vi "Steuerprogramm-15-07-17.vi"() -> ()   [LabVIEW 2010]
uses:
  Emil/Licor-Steuerung/HAGAR V/Licor-Steuerung/display/GUI_Cluster_sdv.ctl
  Emil/Licor-Steuerung/HAGAR V/Licor-Steuerung/display/GUI_Cluster_Parameter.ctl
  Emil/Licor-Steuerung/HAGAR V/Licor-Steuerung/control/Licor-Commands.ctl
  Emil/Licor-Steuerung/HAGAR V/Licor-Steuerung/control/Licor-Parameter.ctl
  Emil/Licor-Steuerung/LicorLI7000/conventions/Licor-Source.ctl
  Emil/Licor-Steuerung/HAGAR V/Licor-Steuerung/control/Licor-Pump.ctl
  Emil/Licor-Steuerung/HAGAR V/Licor-Steuerung/display/GUI_Cluster_Graph.ctl
  Emil/Licor-Steuerung/HAGAR V/Licor-Steuerung/control/Licor-Sequences.ctl
  <vilib>/rvi/interface/nirviMethod/nirviMethod.xnode
  C:/Users/HAGAR-IV/Desktop/Zeugs/markus/version feb 2012/FPGA Bitfiles/pertrasgcfpga2_FPGATarget_FPGA-Programm-05_A75D3647.lvbitx
  C:/Users/HAGAR-IV/Desktop/Zeugs/Johnny/pertrasgc fpga/FPGA-Programm-05-17.vi
  <vilib>/rvi/interface/common/niFpgaNodeNameForErrorReporting.ctl
  <vilib>/rvi/errors/niLvFpgaWhatHappensToTopLevelVI.ctl
  <vilib>/rvi/interface/nirviReadWriteControl/nirviReadWriteControl.xnode
  <vilib>/rvi/interface/nirviCloseFPGA/nirviCloseFPGA.xnode
  GVProbenvol.vi
  GVZeitenZyklen.vi
  GVECDs.vi
  GVZwangs.vi
  GVMethodenwechsel.vi
  GVTrapsMachs.vi
  GVHK1Hz.vi
  GVAIs.vi
  gvbooleschRT.vi
  GVMetavariablen.vi
  GVVentilposition.vi
  GVHorstSP.vi
  GVMWHorst.vi
  GVHeizenLH.vi
  <vilib>/Utility/error.llb/Error Cluster From Error Code.vi
  <vilib>/rvi/errors/niLvFpgaAdjustHostInterfaceError.vi
  GVaktuelleTDMS.vi
  Emil/Licor-Steuerung/HAGAR V/Licor-Steuerung/control/Emulate Licor output GV.vi
  GVChroms.vi
  GVZwangsMPV.vi
  <vilib>/FPGAPlugInAG/cRIO-9114/niLvFpga_Close_cRIO-9114.vi
  NiFpgaLv.dll
  Emil/Licor-Steuerung/HAGAR V/Licor-Steuerung/Licor-Steuerung.lvlib
  <vilib>/NI_Real-Time Target Support.lvlib
  Emil/Licor-Steuerung/LicorLI7000/LicorLI7000.lvlib
panel:
  in  "Zyklus":enum16{"Mod0", "Mod1", "Mod2A", "Mod2B"}(ring)=enum."Mod1"
  in  "am Ende benutzen":bool
  in  "Methode speichern":bool
  out "ZyklusNummernGesamt":i32[](array[numeric])
  in  "veränderte Methode benutzen":bool
  in  "Methode verändern":bool
  out "ZyklusNummern":i32[](array[numeric])
  out "Big Ben, Methodenzeit, Zykluszeit0, Zykluszeit1, Zykluszeit2A, Zykluszeit2B":i32[](array[numeric])
  in  "global stop RT":bool
  in  "Methode":i32(ring) items=["Bedingsmethode", "Startmethode", "Meßmodus", "Shut-up-Methode", "Test", "HAG2 1/2", "Startmethode", "HAG2 1/2 Aufwärmen", "LicorDruckProfil1", "LicorDruckProfil2", "LicorDruckProfil0", "LicorDruckProfil3", "Kalibration-Meßmodus", "Kalibration-Meßmodus-II", "Kalibration-MesmodusIII", "Kalibration-Messmodus-IV", "Kalibration-ECD", "", "Kalibration-ECD-Blank", "Linearitätstest MS"]
  in  "Registerkarte":T1(tab)
  out "SHOK?":bool[](array[boolean])
  out "schnelle Heizungen":string[](array[string])
  out "schnelle Heizungen":dbl[](array[numeric])
  out "HorstOK?":bool[](array[boolean])
  out "AIs3OK?":bool[](array[boolean])
  out "AIs1OK?":bool[](array[boolean])
  out "AIs1":dbl[](array[numeric])
  out "AIs1":string[](array[string])
  out "AIs2":string[](array[string])
  out "AIs3":string[](array[string])
  out "AIs2":dbl[](array[numeric])
  out "AIs3":dbl[](array[numeric])
  out "Metavariablen":string[](array[string])
  out "MVWerte":dbl[](array[numeric])
  out "MWHorst":dbl[](array[numeric])
  out "HorstRegler":string[](array[string])
  out "AIs2OK?":bool[](array[boolean])
  out "Ventilposition":i32=1 min=1 max=6 step=1
  out "MVOK?":bool[](array[boolean])
  out "CPU Total (%)":dbl
  in  "MVFixwert":dbl[](array[numeric])
  in  "MVFix?":bool[](array[boolean])
  in  "LH-Gruppe":bool[](array[boolean])=[FALSE, FALSE, FALSE, FALSE, FALSE, FALSE, FALSE, FALSE, FALSE, FALSE, FALSE, FALSE]
  out "LangsameHeizungen":string[](array[string])
  out "Housekeeping1":cluster{dbl[], dbl[]}(graph)
  in  "Zeitachse1":i32(ring)=1 items=["Zykluszeit [s] Mod0", "Zykluszeit [s] Mod1", "Zykluszeit [s] Mod2A", "Zykluszeit [s] Mod2B"]
  in  "dargestellte Größe 1":i32(ring)=1 items=["T1-Spare1", "T1-Spare2", "T1-StirlingKühlkopf [°C]", "T1-PreCol1 [°C]", "T1-PreCol2 [°C]", "T1-MainCol1a [°C]", "T1-MainCol1b [°C]", "T1-MainCol2a [°C]", "T1-MainCol2b [°C]", "T1-BronkhorstUntena [°C]", "T1-BronkhorstUntenb [°C]", "T1-BronkhorstObena [°C]", "T1-BronkhorstObenb [°C]", "T1-2Pos1B [°C]", "T1-Spare9", "T1-2Pos1A [°C]", "T1-Spare10", "T1-TurboPump [°C]", "T1-StirlingPlatine [°C]", "T1-Spare5", "T1-Spare6", "T1-Spare7", "T1-Inlet [°C]", "F1-MFM-Spare", "F1-MFM0D [mL]", "P1-HeliumHP [bara]", "P1-HeliumLP [bara]", "P1-PumpVordruck [mbara]", "TurboSpeed", "I1-MS-AC [A]", "I1-Trap1 [A]", "I1-Trap2 [A]", "T2-ECD1a", "T2-ECD1b", "T2-ECD2a", "T2-ECD2b", "T2-Col1a", "T2-Col1b", "T2-Col2a", "T2-Col2b", "T2-Spare1", "T2-Spare2", "T2-Spare3", "T2-Spare4", "T2-Spare5", "T2-Spare6", "T2-Spare7", "F2-MFM2A", "F2-MFM2B", "F2-MFM2C", "P2-N2O_HP", "P2-N2O_LP", "P2-CO2_HP", "P2-CO2_LP", "AI-Spare1", "FL-MFM1000mL", "AI-Spare3", "AI-Spare4", "StirlingAlarm", "StirlingEmerg.", "AI-Spare7", "AI-Spare8", "AI-Spare9", "FL-MFM30mL", "T0-DC/DC5", "I0-24V_M0", "I0-48V_M1", "I0-24V_M1", "I0-28V_M2", "T0-Spare3", "T0-Spare2", "T0-Spare4", "T0-DC/DC7", "I0-20V_Laptop", "I0-28V_M1", "I0-24V_M2", "I0-12V_Licor", "T0-Spare1", "T0-Drier", "T0-Spare5", "F0-MFM0A [L]", "TL-Licor_a", "P0-Span-HP", "P0-spare1", "P0-Stickstoff-LP", "P0-Helium-LP", "P0-Cal-HP", "P0-P9Tavco[bar]", "F0-MFM0B [L]", "TL-Licor_b", "P0-Span-LP", "P0-spare2", "P0-Stickstoff-HP", "P0-Helium-HP", "P0-Cal-LP", "F0-MFM3", "Trap1 [°C]", "Trap2 [°C]", "PreCol1 [°C]", "PreCol2 [°C]", "MainCol1 [°C]", "MainCol2 [°C]", "PrC0 [bara]", "PrC0-Licor [bara]", "PrC1-Säule1 [bara]", "PrC1-Säule2 [bara]", "MFC1-Sample [ml/min]", "PrC1-BackFlush1 [bara]", "PrC1-BackFlush2 [bara]", "MFC1-Reaktant [l/min]", "MFC2A[ml/min]", "MFC2B[ml/min]", "MFC2C[ul/min]", "PrC2A[bara]", "MFC2D[ml/min]", "MFC2E[ml/min]", "PrC2B[bara]"]
  out "Housekeeping2":cluster{dbl[], dbl[]}(graph)
  in  "Zeitachse2":i32(ring)=1 items=["Zykluszeit [s] Mod0", "Zykluszeit [s] Mod1", "Zykluszeit [s] Mod2A", "Zykluszeit [s] Mod2B"]
  in  "dargestellte Größe 2":i32(ring)=1 items=["T1-Spare1", "T1-Spare2", "T1-StirlingKühlkopf [°C]", "T1-PreCol1 [°C]", "T1-PreCol2 [°C]", "T1-MainCol1a [°C]", "T1-MainCol1b [°C]", "T1-MainCol2a [°C]", "T1-MainCol2b [°C]", "T1-BronkhorstUntena [°C]", "T1-BronkhorstUntenb [°C]", "T1-BronkhorstObena [°C]", "T1-BronkhorstObenb [°C]", "T1-2Pos1B [°C]", "T1-Spare9", "T1-2Pos1A [°C]", "T1-Spare10", "T1-TurboPump [°C]", "T1-StirlingPlatine [°C]", "T1-Spare5", "T1-Spare6", "T1-Spare7", "T1-Inlet [°C]", "F1-MFM-Spare", "F1-MFM0D [mL]", "P1-HeliumHP [bara]", "P1-HeliumLP [bara]", "P1-PumpVordruck [mbara]", "TurboSpeed", "I1-MS-AC [A]", "I1-Trap1 [A]", "I1-Trap2 [A]", "T2-ECD1a", "T2-ECD1b", "T2-ECD2a", "T2-ECD2b", "T2-Col1a", "T2-Col1b", "T2-Col2a", "T2-Col2b", "T2-Spare1", "T2-Spare2", "T2-Spare3", "T2-Spare4", "T2-Spare5", "T2-Spare6", "T2-Spare7", "F2-MFM2A", "F2-MFM2B", "F2-MFM2C", "P2-N2O_HP", "P2-N2O_LP", "P2-CO2_HP", "P2-CO2_LP", "AI-Spare1", "FL-MFM1000mL", "AI-Spare3", "AI-Spare4", "StirlingAlarm", "StirlingEmerg.", "AI-Spare7", "AI-Spare8", "AI-Spare9", "FL-MFM30mL", "T0-DC/DC5", "I0-24V_M0", "I0-48V_M1", "I0-24V_M1", "I0-28V_M2", "T0-Spare3", "T0-Spare2", "T0-Spare4", "T0-DC/DC7", "I0-20V_Laptop", "I0-28V_M1", "I0-24V_M2", "I0-12V_Licor", "T0-Spare1", "T0-Drier", "T0-Spare5", "F0-MFM0A [L]", "TL-Licor_a", "P0-Span-HP", "P0-spare1", "P0-Stickstoff-LP", "P0-Helium-LP", "P0-Cal-HP", "P0-P9Tavco[bar]", "F0-MFM0B [L]", "TL-Licor_b", "P0-Span-LP", "P0-spare2", "P0-Stickstoff-HP", "P0-Helium-HP", "P0-Cal-LP", "F0-MFM3", "Trap1 [°C]", "Trap2 [°C]", "PreCol1 [°C]", "PreCol2 [°C]", "MainCol1 [°C]", "MainCol2 [°C]", "PrC0 [bara]", "PrC0-Licor [bara]", "PrC1-Säule1 [bara]", "PrC1-Säule2 [bara]", "MFC1-Sample [ml/min]", "PrC1-BackFlush1 [bara]", "PrC1-BackFlush2 [bara]", "MFC1-Reaktant [l/min]", "MFC2A[ml/min]", "MFC2B[ml/min]", "MFC2C[ul/min]", "PrC2A[bara]", "MFC2D[ml/min]", "MFC2E[ml/min]", "PrC2B[bara]"]
  out "Detektor 2":cluster{dbl[], dbl[]}[](graph)
  in  "Detektor":i32(ring) items=["ECD1", "ECD2"]
  in  "HK1YMin":dbl
  in  "HK1YMax":dbl=100.0
  in  "HK2YMin":dbl
  in  "HK2YMax":dbl=100.0
  in  "DetYMin":dbl
  in  "DetYMax":dbl=100.0
  in  "NeuerRefstrom":bool
  in  "RefStromECD1":i16=800 min=0 max=2500 step=1
  in  "RefStromECD2":i16=2100 min=0 max=2500 step=1
  out "schnelleAnzeige":cluster{dbl[], dbl[]}(graph)
  in  "TafelWischen!":bool
  in  "dargestellte Größe 3":i32(ring)=1 items=["Trap1 [°C]", "Trap2 [°C]", "PreCol1 [°C]", "PreCol2 [°C]", "MainCol1 [°C]", "MainCol2 [°C]", "PrC0 [bara]", "PrC0-Licor [bara]", "PrC1-Säule1 [bara]", "PrC1-Säule2 [bara]", "MFC1-Sample [ml/min]", "PrC1-BackFlush1 [bara]", "PrC1-BackFlush2 [bara]", "MFC1-Reaktant [l/min]", "MFC2A[ml/min]", "MFC2B[ml/min]", "MFC2C[ul/min]", "PrC2A[bara]", "MFC2D[ml/min]", "MFC2E[ml/min]", "PrC2B[bara]"]
  in  "An/Aus":bool
  in  "Registerkarte 2":T2(tab)
  in  "GUI_Cluster_Graph":T3={"time (global)"=0.0, "command queue"=[], "Rohdaten"=[], "Graph"={"X"=[], "Y"=[]}, "Manuelle Steuerung"={"Sequenz"=enum."test", "Manuelle Steuerung An/Aus"=FALSE}, "Sequenz out"={"sequence"=enum."WAIT", "Zeitpunkt next"=0.0, "delta t"=0.0}} caption="Cluster" {"Sequenz out"."Zeitpunkt next" format="%<%H:%M:%S%3u>T"; "time (global)" format="%<%H:%M:%S%3u\n%m/%d/%y>T"}
  in  "GUI_Cluster_Parameter":T5={"warmup (sequence)"=[{"time"=60, "Enum"=enum."wait"}], "calibrate S (sequence)"=[{"time"=60, "Enum"=enum."wait"}, {"time"=2, "Enum"=enum."getCalibrationParameter"}, {"time"=8, "Enum"=enum."calibration-S-CO2"}, {"time"=2, "Enum"=enum."getCalibrationParameter"}], "calibrate Z (sequence)"=[{"time"=60, "Enum"=enum."wait"}, {"time"=2, "Enum"=enum."getCalibrationParameter"}, {"time"=8, "Enum"=enum."calibration-Z-H2O"}, {"time"=2, "Enum"=enum."getCalibrationParameter"}, {"time"=8, "Enum"=enum."calibration-Z-CO2"}, {"time"=2, "Enum"=enum."getCalibrationParameter"}], "initialize (sequence)"=[{"time"=30, "Enum"=enum."wait"}, {"time"=2, "Enum"=enum."setPumpSlow"}, {"time"=2, "Enum"=enum."setPumpMedium"}, {"time"=2, "Enum"=enum."setPumpFast"}, {"time"=10, "Enum"=enum."initialize"}, {"time"=4, "Enum"=enum."getCalibrationParameter"}, {"time"=2, "Enum"=enum."resetH2O"}, {"time"=4, "Enum"=enum."resetCO2"}, {"time"=4, "Enum"=enum."getCalibrationParameter"}, {"time"=2, "Enum"=enum."setZeroParameter"}, {"time"=4, "Enum"=enum."getCalibrationParameter"}, {"time"=2, "Enum"=enum."setReference"}, {"time"=4, "Enum"=enum."getLicorTime"}, {"time"=5, "Enum"=enum."getInfo"}], "Licor-parameter"={"CO2 ref"=378.15, "CO2 span"=401.67, "H2O ref"=0.0, "H2O span"=0.0, "Zi"=1.2, "Zt"=6.494e-05, "Zm"=0.0, "S"=1.34, "Temp [C]"=45.0, "Pressure [hPa]"=1050.0, "Licor-Sources"=["CO2A W", "CO2B W", "H2OA W", "H2OB W", "T C", "T V", "P kPa", "P V", "RH %"], "Licor-Pump"="Off", "Zeitstempel"=timestamp(0 s since 1904-01-01)}} {"Licor-parameter"."Pressure [hPa]" format="%_5g"; "Licor-parameter"."Temp [C]" format="%.2f"; "Licor-parameter"."CO2 ref" format="%.2f"; "Licor-parameter"."CO2 span" format="%.2g"; "Licor-parameter"."H2O ref" format="%.2g"; "Licor-parameter"."H2O span" format="%.2g"; "Licor-parameter"."Zt" format="%#_4g"}
  in  "GUI_Cluster_sdv":T10={"Graph_sdv"={"X"=[], "Y"=[]}, "Breite"=20, "Berechnen"=FALSE, "residue"=0.0} {"residue" format="%_6g"}
  in  "VISA resource name":refnum<visa-resource-name>="ASRL1::INSTR" caption="VISA-Ressourcenname"
  out "TDMSwriteECD":errorcluster
  out "AIsFIFOread":errorcluster
  out "MWTrapsMachs":errorcluster
  out "TDMSwriteHK":errorcluster
  out "TDMScloseHK":errorcluster
  out "TDMSopenHK":errorcluster
  out "TDMScloseECD2":errorcluster
  out "TDMSopenECD2":errorcluster
  out "TDMScloseECD1":errorcluster
  out "TDMSopenECD1":errorcluster
  out "FIFOwriteRS485":errorcluster
  out "SerielleKomm.":errorcluster
  out "LH":errorcluster
  out "Zyklus":errorcluster
  out "ECD1dataBackup":errorcluster
  out "ECD2dataBackup":errorcluster
  # "Zyklen:   ===>>"
  # "MS"
  # "ECD1"
  # "ECD2"
  # "Zykluszeiten:   ===>>"
  # "MS"
  # "ECD1"
  # "ECD2"
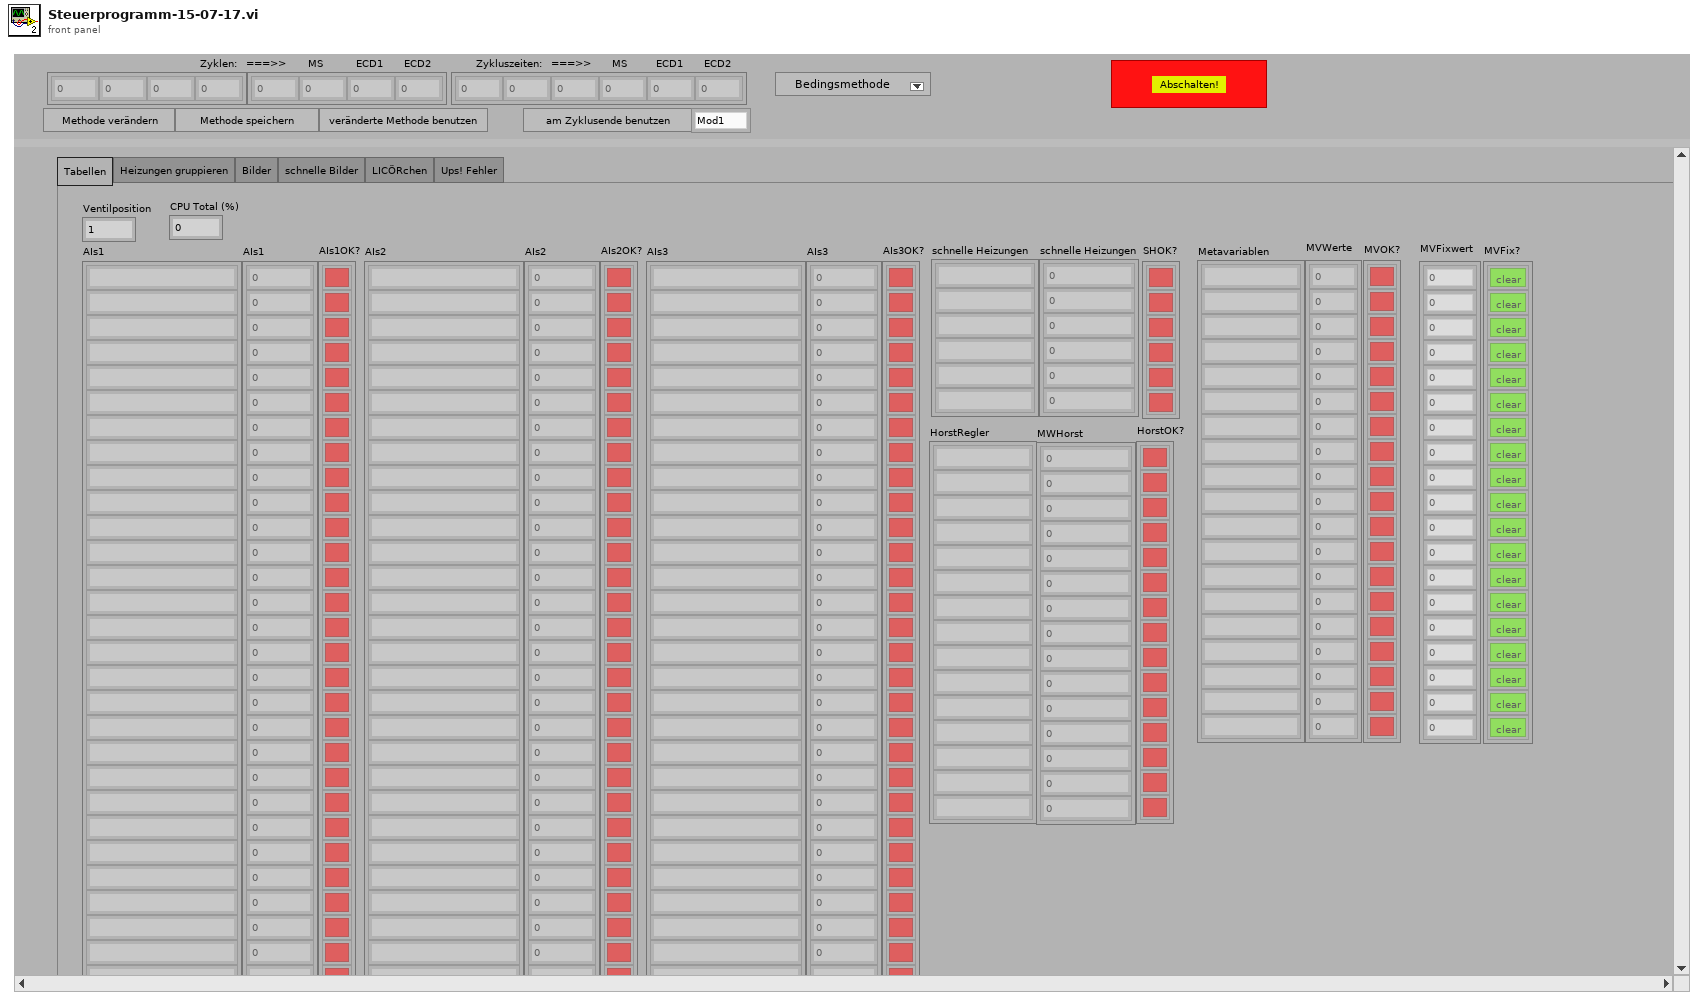
[diagram p1: front panel]
types:
  T1 = enum32{"Tabellen", "Heizungen gruppieren", "Bilder", "schnelle Bilder", "LICÖRchen", "Ups! Fehler"}
  T2 = enum32{"Graph", "Parameter / Sequenzen", "sdv", "debug"}
  T3 = typedef "Licor-Steuerung.lvlib/GUI_Cluster_Graph.ctl" = cluster{"time (global)":dbl, "command queue":cluster{"Zeit [s]":i32, "Befehl":string}[], "Rohdaten":string[], "Graph":cluster{"X":dbl[], "Y":dbl[]}, "Manuelle Steuerung":cluster{"Sequenz":T4, "Manuelle Steuerung An/Aus":bool}, "Sequenz out":cluster{"sequence":T4, "Zeitpunkt next":dbl, "delta t":dbl}}
  T4 = typedef "Licor-Steuerung.lvlib/Licor-Sequences.ctl" = enum16{"test", "WAIT", "warmup", "initialize", "calibrate Z", "calibrate S"}
  T5 = typedef "Licor-Steuerung.lvlib/GUI_Cluster_Parameter.ctl" = cluster{"warmup (sequence)":cluster{"time":i32, "Enum":T6}[], "calibrate S (sequence)":cluster{"time":i32, "Enum":T6}[], "calibrate Z (sequence)":cluster{"time":i32, "Enum":T6}[], "initialize (sequence)":cluster{"time":i32, "Enum":T6}[], "Licor-parameter":T7}
  T6 = typedef "Licor-Steuerung.lvlib/Licor-Commands.ctl" = enum16{"wait", "initialize", "resetCO2", "resetH2O", "getReference", "setReference", "calibration-Z-CO2", "calibration-Z-H2O", "calibration-S-CO2", "calibration-S-H2O", "getCalibrationParameter", "setZeroParameter", "setLicorTime", "getLicorTime", "setPumpFlowrate", "setPumpSlow", "setPumpMedium", "setPumpFast", "getInfo"}
  T7 = typedef "Licor-Steuerung.lvlib/Licor-Parameter.ctl" = cluster{"CO2 ref":dbl, "CO2 span":dbl, "H2O ref":dbl, "H2O span":dbl, "Zi":dbl, "Zt":dbl, "Zm":dbl, "S":dbl, "Temp [C]":dbl, "Pressure [hPa]":dbl, "Licor-Sources":T8[], "Licor-Pump":T9, "Zeitstempel":timestamp}
  T8 = typedef "LicorLI7000.lvlib/Licor-Source.ctl" = string
  T9 = typedef "Licor-Steuerung.lvlib/Licor-Pump.ctl" = string
  T10 = typedef "Licor-Steuerung.lvlib/GUI_Cluster_sdv.ctl" = cluster{"Graph_sdv":cluster{"X":dbl[], "Y":dbl[]}, "Breite":i32, "Berechnen":bool, "residue":dbl}
  T11 = cluster{"Zykluslängen [s]":dbl[], "ZeitpktDIOsMod0":dbl[], "ZeitpktDIOsMod1":dbl[], "ZeitpktDIOsMod2A":dbl[], "ZeitpktDIOsMod2B":dbl[], "DIOsSPMod0":bool[][], "DIOsSPMod1":bool[][], "DIOsSPMod2A":bool[][], "DIOsSPMod2B":bool[][], "Mod0HorstZeitpkt":dbl[], "Mod1HorstZeitpkt":dbl[], "Mod2AHorstZeitpkt":dbl[], "Mod2BHorstZeitpkt":dbl[], "HorstSPMod0":dbl[][], "HorstSPMod1":dbl[][], "HorstSPMod2A":dbl[][], "HorstSPMod2B":dbl[][], "LHSetpoints":dbl[], "LHHeizen?":bool[], "ZPktFPGABoolesch":dbl[], "FPGABoolesch":bool[][], "ZeitpktFPGAPID":dbl[], "FPGAPID":cluster{"d0":fxp<+/-,18,18>, "d1":fxp<+/-,21,21>}[][], "ZeitpktFPGAFixp":dbl[], dbl[][], "t_PreMach1":dbl[], "T_PreMach1":dbl[], "t_PreMach2":dbl[], "T_PreMach2":dbl[], "PIDs für \"träge\" Heizungen":cluster{"proportional gain (Kc)":dbl, "integral time (Ti, min)":dbl, "derivative time (Td, min)":dbl}[], "Zwangsbedingungen":dbl[][], "Dateien fürs MS schicken?":bool, "ZeitpunkteMPV":dbl[], "SPMPV":i32[], "ZeitpktMS-1":dbl, "ZeitpktMS-2":dbl, "Int.Start1":dbl, "Int.Stop1":dbl, "Int.Start2":dbl, "Int.Stop2":dbl, "Methodenname":string, "t_MainMach1":dbl[], "T_MainMach1":dbl[], "t_MainMach2":dbl[], "T_MainMach2":dbl[]}[]
  T12 = cluster{"DIOsMod0Nr":i32[], "DIOsMod1Nr":i32[], "DIOsMod2ANr":i32[], "DIOsMod2BNr":i32[], "AIsLH":i32[], "AnzahlRegler/Modul":i32[], "Regler für den Probenfluß":i32, "SPvorgebenMod0":string[], "SPvorgebenMod1":string[], "SPvorgebenMod2A":string[], "SPvorgebenMod2B":string[], "MWAntwortMod0":string[], "MWAntwortMod1":string[], "MWAntwortMod2A":string[], "MWAntwortMod2B":string[], "FaktorMod0":dbl[], "FaktorMod1":dbl[], "FaktorMod2A":dbl[], "FaktorMod2B":dbl[], "MWabfragenMod0":string[], "MWabfragenMod1":string[], "MWabfragenMod2A":string[], "MWabfragenMod2B":string[], "Modul1/AI koeff":dbl[][], "Modul2/AI koeff":dbl[][], "Modul3/AI koeff":dbl[][], "Traps/MachsKoeff T(R)":dbl[][], "Modul1/AIsNamen":string[], "Modul2/AIsNamen":string[], "Modul3/AIsNamen":string[], "DIOsMod0Name":string[], "DIOsMod1Name":string[], "DIOsMod2AName":string[], "DIOsMod2BName":string[], "ReglerNameMod0":string[], "ReglerNameMod1":string[], "ReglerNameMod2A":string[], "ReglerNameMod2B":string[], "Startmethode":i32, "Dateiordner Housekeeping":path, "Dateiname Housekeeping":string, "DateiordnerECD1":path, "DateinameECD1":string, "DateiordnerECD2":path, "DateinameECD2":string, "LangsameHeizungen":string[], "ModuleLH":i32[], "Metavariablen":string[], "Modul1/AI sicherer Bereich":dbl[][], "Modul2/AI sicherer Bereich":dbl[][], "Modul3/AI sicherer Bereich":dbl[][], "Traps/Machs sicherer Bereich":dbl[][], "ReglerMod0 sicherer Bereich":dbl[][], "ReglerMod1 sicherer Bereich":dbl[][], "ReglerMod2A sicherer Bereich":dbl[][], "ReglerMod2B sicherer Bereich":dbl[][], "Metavariablen grüner Bereich":dbl[][], "Traps/MachsKoeff R(U)":dbl[][], "LHGruppe":bool[]}
  T13 = enum16{"open", "replace", "create", "open or create", "replace or create", "replace or create with confirmation"}
  T14 = typedef "niFpgaNodeNameForErrorReporting.ctl" = enum16{"Open FPGA VI Reference", "Read/Write Control", "Invoke Method: Abort", "Invoke Method: Acknowledge IRQ", "Invoke Method: Download", "Invoke Method: FIFO.Configure", "Invoke Method: FIFO.Read", "Invoke Method: FIFO.Start", "Invoke Method: FIFO.Stop", "Invoke Method: FIFO.Write", "Invoke Method: Reset", "Invoke Method: Run", "Invoke Method: Wait on IRQ", "Close FPGA VI Reference"}
  T15 = typedef "niLvFpgaWhatHappensToTopLevelVI.ctl" = enum16{"top level VI scripted behind XNode", "top level VI inlined behind XNode"}
  T16 = cluster{"Zyklus1":i32, "Zeitachse1":i32, "dargestellte Größe 1":i32, "Zyklus2":i32, "Zeitachse2":i32, "dargestellte Größe 2":i32}
  T17 = cluster{"DIOsMod0Name":string[], "DIOsMod1Name":string[], "DIOsMod2AName":string[], "DIOsMod2BName":string[], "ReglerNameMod0":string[], "ReglerNameMod1":string[], "ReglerNameMod2A":string[], "ReglerNameMod2B":string[], "LangsameHeizungen":string[]}
  T18 = cluster{"Zykluslängen [s]":dbl[], "ZeitpktDIOsMod0":dbl[], "ZeitpktDIOsMod1":dbl[], "ZeitpktDIOsMod2A":dbl[], "ZeitpktDIOsMod2B":dbl[], "DIOsSPMod0":bool[][], "DIOsSPMod1":bool[][], "DIOsSPMod2A":bool[][], "DIOsSPMod2B":bool[][], "Mod0HorstZeitpkt":dbl[], "Mod1HorstZeitpkt":dbl[], "Mod2AHorstZeitpkt":dbl[], "Mod2BHorstZeitpkt":dbl[], "HorstSPMod0":dbl[][], "HorstSPMod1":dbl[][], "HorstSPMod2A":dbl[][], "HorstSPMod2B":dbl[][], "LHSetpoints":dbl[], "LHHeizen?":bool[], "ZPktFPGABoolesch":dbl[], "FPGABoolesch":bool[][], "ZeitpktFPGAPID":dbl[], "FPGAPID":cluster{"d0":fxp<+/-,18,18>, "d1":fxp<+/-,21,21>}[][], "ZeitpktFPGAFixp":dbl[], dbl[][], "t_PreMach1":dbl[], "T_PreMach1":dbl[], "t_PreMach2":dbl[], "T_PreMach2":dbl[], "PIDs für \"träge\" Heizungen":cluster{"proportional gain (Kc)":dbl, "integral time (Ti, min)":dbl, "derivative time (Td, min)":dbl}[], "Zwangsbedingungen":dbl[][], "Dateien fürs MS schicken?":bool, "ZeitpunkteMPV":dbl[], "SPMPV":i32[], "ZeitpktMS-1":dbl, "ZeitpktMS-2":dbl, "Int.Start1":dbl, "Int.Stop1":dbl, "Int.Start2":dbl, "Int.Stop2":dbl, "Methodenname":string, "t_MainMach1":dbl[], "T_MainMach1":dbl[], "t_MainMach2":dbl[], "T_MainMach2":dbl[]}
  T19 = cluster{"Modul1/AI sicherer Bereich":dbl[][], "Modul2/AI sicherer Bereich":dbl[][], "Modul3/AI sicherer Bereich":dbl[][], "Traps/Machs sicherer Bereich":dbl[][], dbl[][], "Metavariablen grüner Bereich":dbl[][]}
  T20 = cluster{"created path":path, "created path":path}
  T21 = cluster{"created path":path, "created path":path, "created path":path, "Dateiname Housekeeping":string, "DateinameECD1":string, "DateinameECD2":string, "tdms0":refnum<k34>, "tdms1":refnum<k34>, "tdms0":refnum<k34>, "tdms1":refnum<k34>, "tdms0":refnum<k34>, "tdms1":refnum<k34>}
  T22 = cluster{"d0":fxp<+/-,18,18>, "d1":fxp<+/-,21,21>}[][]
  T23 = cluster{"proportional gain (Kc)":dbl, "integral time (Ti, min)":dbl, "derivative time (Td, min)":dbl}[]
  T24 = cluster{cluster{"ZeitpktDIOsMod2B":dbl[]}[], cluster{"DIOsSPMod2B":bool[][]}[], cluster{"Mod2BHorstZeitpkt":dbl[]}[], cluster{"HorstSPMod2B":dbl[][]}[], "LHHeizen?":bool[], "ZPktFPGABoolesch":dbl[], "FPGABoolesch":bool[][], "ZeitpktFPGAPID":dbl[], "FPGAPID":cluster{"d0":fxp<+/-,18,18>, "d1":fxp<+/-,21,21>}[][], "ZeitpktFPGAFixp":dbl[], dbl[][], "t_PreMach1":dbl[], "T_PreMach1":dbl[], "t_PreMach2":dbl[], "T_PreMach2":dbl[], "ZeitpunkteMPV":dbl[], "SPMPV":i32[], "t_MainMach1":dbl[], "T_MainMach1":dbl[], "t_MainMach2":dbl[], "T_MainMach2":dbl[]}
  T25 = cluster{"Zykluslängen [s]":dbl[], "ZeitpktDIOsMod0":dbl[], "ZeitpktDIOsMod1":dbl[], "ZeitpktDIOsMod2A":dbl[], "ZeitpktDIOsMod2B":dbl[], "DIOsSPMod0":bool[][], "DIOsSPMod1":bool[][], "DIOsSPMod2A":bool[][], "DIOsSPMod2B":bool[][], "Mod0HorstZeitpkt":dbl[], "Mod1HorstZeitpkt":dbl[], "Mod2AHorstZeitpkt":dbl[], "Mod2BHorstZeitpkt":dbl[], "HorstSPMod0":dbl[][], "HorstSPMod1":dbl[][], "HorstSPMod2A":dbl[][], "HorstSPMod2B":dbl[][], "LangsameHeizungenSP":dbl[], "LHHeizen?":bool[], "ZPktFPGABoolesch":dbl[], "FPGABoolesch":bool[][], "ZeitpktFPGAPID":dbl[], "FPGAPID":cluster{"d0":fxp<+/-,18,18>, "d1":fxp<+/-,21,21>}[][], "ZeitpktFPGAFixp":dbl[], "FPGAFixp":dbl[][], "t_PreMach1":dbl[], "T_PreMach1":dbl[], "t_PreMach2":dbl[], "T_PreMach2":dbl[], "PIDs für \"träge\" Heizungen":cluster{"proportional gain (Kc)":dbl, "integral time (Ti, min)":dbl, "derivative time (Td, min)":dbl}[], "Zwangsbedingungen":dbl[][], "MS-Daten?":bool, "ZeitpunkteMPV":dbl[], "SetpointMPV":i32[], "ZeitpktMS-1":dbl, "ZeitpktMS-2":dbl, "Int.Start1":dbl, "Int.Stop1":dbl, "Int.Start2":dbl, "Int.Stop2":dbl, "Methodenname":string, "t_MainMach1":dbl[], "T_MainMach1":dbl[], "t_MainMach2":dbl[], "T_MainMach2":dbl[]}
  T26 = cluster{"ZyklusNummern":i32[], "ZeilennummernDIOs":i32[], "ZwangsDIO?":cluster{bool[]}[], "ZeilennummernHorst":i32[], "ZwangsHorst?":cluster{bool[]}[], "ZeileFPGABoolesch":i32, "ZwangsFPGABoolesch?":bool[], "ZeileFPGAPID":i32, "ZeileFPGAFixp":i32, "ZeilePreMach1":i32, "ZeilePreMach2":i32, "ZeilennummerMPV":i32, "ZeileMainMach1":i32, "ZeileMainMach2":i32, "ZwangsMPV?":bool}
  T27 = typedef "NI_Real-Time Target Support.lvlib/RT CPU Load.ctl" = cluster{"Total (%)":dbl, "Time Critical (%)":dbl, "Timed Structures (%)":dbl, "High (%)":dbl, "Above Normal (%)":dbl, "Normal (%)":dbl, "Background (%)":dbl, "Idle (%)":dbl, "ISR (%)":dbl}
  T28 = cluster{"ZyklusNummern":i32[], i32[], "ZwangsDIO?":cluster{bool[]}[], i32[], "ZwangsHorst?":cluster{bool[]}[], i32, "ZwangsFPGABoolesch?":bool[], i32, i32, "ZeileMach":i32, "ZeileMach":i32, i32, "ZeileMach":i32, "ZeileMach":i32, "ZwangsMPV?":bool}
  T29 = cluster{string[], string[], string[], dbl[], dbl[], dbl[]}
  T30 = cluster{"Befehle1":string[], "Befehle2":string[], "Befehle3":string[]}
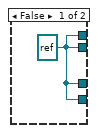
[diagram p2: hidden frame]
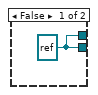
[diagram p3: hidden frame]
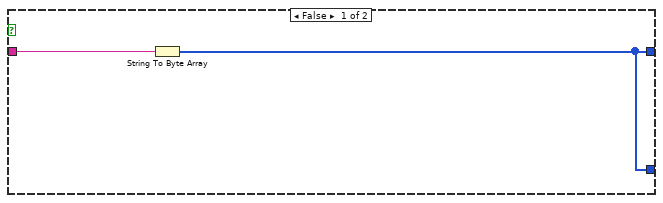
[diagram p6: hidden frame]
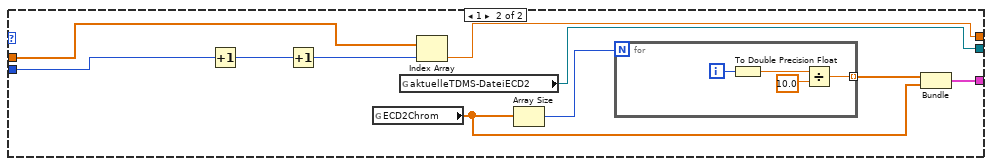
[diagram p16: hidden frame]
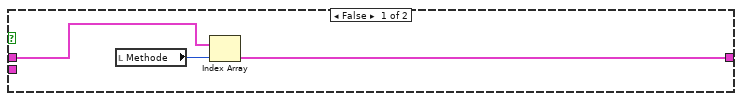
[diagram p17: hidden frame]
diagram:
  w2 = path "c:/methoden.pery" ("Datei (Dialog verwenden)")
  w3 = path "c:/einstellungen.pery" ("Datei (Dialog verwenden)")
  n1 = Open/Create/Replace File(file path (use dialog)=w3, operation (0:open)=T13."open" ("Operation (0:Öffnen)")) -> (refnum out=w15:refnum<file>)  [unwired: 4 in, 2 out]
  n2 = Open/Create/Replace File(file path (use dialog)=w2, operation (0:open)=T13."open" ("Operation (0:Öffnen)")) -> (refnum out=w11:refnum<file>)  [unwired: 4 in, 2 out]
  n3 = Read from Binary File(5:T12 {"DIOsMod0Nr"=[], "DIOsMod1Nr"=[], "DIOsMod2ANr"=[], "DIOsMod2BNr"=[], "AIsLH"=[], "AnzahlRegler/Modul"=[], "Regler für den Probenfluß"=0, "SPvorgebenMod0"=[], "SPvorgebenMod1"=[], "SPvorgebenMod2A"=[], "SPvorgebenMod2B"=[], "MWAntwortMod0"=[], "MWAntwortMod1"=[], "MWAntwortMod2A"=[], "MWAntwortMod2B"=[], "FaktorMod0"=[], "FaktorMod1"=[], "FaktorMod2A"=[], "FaktorMod2B"=[], "MWabfragenMod0"=[], "MWabfragenMod1"=[], "MWabfragenMod2A"=[], "MWabfragenMod2B"=[], "Modul1/AI koeff"=[], "Modul2/AI koeff"=[], "Modul3/AI koeff"=[], "Traps/MachsKoeff T(R)"=[], "Modul1/AIsNamen"=[], "Modul2/AIsNamen"=[], "Modul3/AIsNamen"=[], "DIOsMod0Name"=[], "DIOsMod1Name"=[], "DIOsMod2AName"=[], "DIOsMod2BName"=[], "ReglerNameMod0"=[], "ReglerNameMod1"=[], "ReglerNameMod2A"=[], "ReglerNameMod2B"=[], "Startmethode"=0, "Dateiordner Housekeeping"=path "", "Dateiname Housekeeping"="", "DateiordnerECD1"=path "", "DateinameECD1"="", "DateiordnerECD2"=path "", "DateinameECD2"="", "LangsameHeizungen"=[], "ModuleLH"=[], "Metavariablen"=[], "Modul1/AI sicherer Bereich"=[], "Modul2/AI sicherer Bereich"=[], "Modul3/AI sicherer Bereich"=[], "Traps/Machs sicherer Bereich"=[], "ReglerMod0 sicherer Bereich"=[], "ReglerMod1 sicherer Bereich"=[], "ReglerMod2A sicherer Bereich"=[], "ReglerMod2B sicherer Bereich"=[], "Metavariablen grüner Bereich"=[], "Traps/MachsKoeff R(U)"=[], "LHGruppe"=[]} ("output cluster"), 11:w15) -> (2:w13:T12, 3:w14:refnum<file>)  [unwired: 4 in, 2 out]
  n4 = Read from Binary File(5:T11 [], 11:w11) -> (2:w9:T11, 3:w10:refnum<file>)  [unwired: 4 in, 2 out]
  n5 = Close File(refnum=w14) -> ()  [unwired: 1 in, 2 out]
  n6 = Close File(refnum=w10) -> ()  [unwired: 1 in, 2 out]
  n7 = flat-sequence {
    tunnel: [w84] -> w42
    tunnel: [w145] -> w41
    tunnel: [w88] -> w39
    tunnel: [w278] -> w38
    tunnel: [w280] -> w37
    tunnel: [w272] -> w36
    tunnel: [w279] -> w35
    tunnel: [w202] -> w34
    tunnel: [w271] -> w33
    tunnel: [w270] -> w32
    tunnel: [w264] -> w31
    tunnel: [w205] -> w30
    tunnel: [w179] -> w29
    tunnel: [w277] -> w28
    tunnel: [w269] -> w27
    tunnel: [w268] -> w26
    tunnel: [w260] -> w25
    tunnel: [w259] -> w24
    tunnel: [w258] -> w23
    tunnel: [w257] -> w22
    tunnel: [w256] -> w21
    tunnel: [w255] -> w20
    tunnel: [w252] -> w19
    tunnel: [w234] -> w18
    tunnel: w13 -> [w127]
    tunnel: [w233] -> w17
    tunnel: w9 -> [w146]
    tunnel: [w145] -> w8
    tunnel: [w127] -> w7
    tunnel: [w96] -> w6
    tunnel: w3 -> [w81]
    tunnel: w2 -> [w77]
    tunnel: [w58] -> w1
    tunnel: w42 -> [w478]
    tunnel: w41 -> [w551]
    tunnel: [w478] -> w40
    tunnel: w39 -> [_]
    tunnel: w38 -> [w509]
    tunnel: w37 -> [w508]
    tunnel: w36 -> [w510]
    tunnel: w35 -> [w507]
    tunnel: w34 -> [w482]
    tunnel: w33 -> [w477]
    tunnel: w32 -> [w474]
    tunnel: w31 -> [w471]
    tunnel: w30 -> [w472]
    tunnel: w29 -> [w475]
    tunnel: w28 -> [w549]
    tunnel: w27 -> [w480]
    tunnel: w26 -> [w550]
    tunnel: w25 -> [w453]
    tunnel: w24 -> [w452]
    tunnel: w23 -> [w451]
    tunnel: w22 -> [w547]
    tunnel: w21 -> [w546]
    tunnel: w20 -> [w545]
    tunnel: w19 -> [w499]
    tunnel: w18 -> [w481]
    tunnel: w17 -> [w470]
    tunnel: w9 -> [w469]
    tunnel: w8 -> [w467]
    tunnel: w7 -> [_]
    tunnel: w6 -> [w446]
    tunnel: w1 -> [w445]
    tunnel: w40 -> [w1479]
    frame #0 {
      w54 = "config" ("string")
      w76 = string[] ["Trap1 [°C]", "Trap2 [°C]", "PreCol1 [°C]", "PreCol2 [°C]", "MainCol1 [°C]", "MainCol2 [°C]"]
      w147 = TRUE
      w161 = 0.0 ("Probenvol.1")
      w168 = dbl[] [-1.0] ("ECD1MW")
      w169 = FALSE ("ECD1Empfangen?")
      w275 = string[] ["Big Ben [s]", "Methodenzeit [s]", "Zykluszeit [s] Mod0", "Zykluszeit [s] Mod1", "Zykluszeit [s] Mod2A", "Zykluszeit [s] Mod2B"]
      w265 = FALSE ("Undefinierte Werte möglich")
      w266 = FALSE ("global stop RT")
      n8 = for {
        tunnel: [w440] -> w273 mode=indexing
        tunnel: w146 -> [w441] mode=indexing
        n9 = Unbundle(w441) -> ("Methodenname"=w440:string)  [unwired: 44 out]
      }
      n10 = Unbundle(w127) -> ("DIOsMod0Nr"=w189:i32[], "DIOsMod1Nr"=w188:i32[], "DIOsMod2ANr"=w187:i32[], "DIOsMod2BNr"=w186:i32[], "AIsLH"=w176:i32[], "AnzahlRegler/Modul"=w179:i32[], "Regler für den Probenfluß"=w233:i32, "SPvorgebenMod0"=w232:string[], "SPvorgebenMod1"=w231:string[], "SPvorgebenMod2A"=w230:string[], "SPvorgebenMod2B"=w229:string[], "MWAntwortMod0"=w228:string[], "MWAntwortMod1"=w227:string[], "MWAntwortMod2A"=w226:string[], "MWAntwortMod2B"=w225:string[], "FaktorMod0"=w224:dbl[], "FaktorMod1"=w223:dbl[], "FaktorMod2A"=w222:dbl[], "FaktorMod2B"=w221:dbl[], "MWabfragenMod0"=w220:string[], "MWabfragenMod1"=w219:string[], "MWabfragenMod2A"=w218:string[], "MWabfragenMod2B"=w217:string[], "Modul1/AI koeff"=w216:dbl[][], "Modul2/AI koeff"=w215:dbl[][], "Modul3/AI koeff"=w214:dbl[][], "Traps/MachsKoeff T(R)"=w213:dbl[][], "Modul1/AIsNamen"=w212:string[], "Modul2/AIsNamen"=w211:string[], "Modul3/AIsNamen"=w210:string[], "DIOsMod0Name"=w125:string[], "DIOsMod1Name"=w126:string[], "DIOsMod2AName"=w124:string[], "DIOsMod2BName"=w123:string[], "ReglerNameMod0"=w138:string[], "ReglerNameMod1"=w137:string[], "ReglerNameMod2A"=w136:string[], "ReglerNameMod2B"=w135:string[], "Startmethode"=w145:i32, "Dateiordner Housekeeping"=w63:path, "Dateiname Housekeeping"=w209:string, "DateiordnerECD1"=w68:path, "DateinameECD1"=w208:string, "DateiordnerECD2"=w60:path, "DateinameECD2"=w207:string, "LangsameHeizungen"=w206:string[], "ModuleLH"=w201:i32[], "Metavariablen"=w140:string[], "Modul1/AI sicherer Bereich"=w100:dbl[][], "Modul2/AI sicherer Bereich"=w99:dbl[][], "Modul3/AI sicherer Bereich"=w98:dbl[][], "Traps/Machs sicherer Bereich"=w97:dbl[][], "ReglerMod0 sicherer Bereich"=w95:dbl[][], "ReglerMod1 sicherer Bereich"=w94:dbl[][], "ReglerMod2A sicherer Bereich"=w93:dbl[][], "ReglerMod2B sicherer Bereich"=w92:dbl[][], "Metavariablen grüner Bereich"=w90:dbl[][], "LHGruppe"=w83:bool[])  [unwired: 1 out]
      "Metavariablen" <- w140
      "LangsameHeizungen" <- w206
      n11 = Initialize Array(0, 4 ("Dimension")) -> (w162:i32[])
      n12 = Initialize Array(0.0 ("Element"), 6 ("Dimension")) -> (w165:dbl[])
      n13 = global write "GVMethodenwechsel.vi" "Methodenwechsel?"(FALSE ("Methodenwechsel?")) -> ()
      n14 = local write "NeuerRefstrom"(FALSE ("NeuerRefstrom")) -> ()
      n15 = global write "GVProbenvol.vi" "Probenvol.1"(w161) -> ()
      n16 = global write "GVProbenvol.vi" "Probenvol.2"(w161) -> ()
      n17 = global write "GVECDs.vi" "ECD1MW"(w168) -> ()
      n18 = global write "GVECDs.vi" "ECD2MW"(w168) -> ()
      n19 = global write "GVECDs.vi" "ECD1Empfangen?"(w169) -> ()
      n20 = global write "GVECDs.vi" "ECD2Empfangen?"(w169) -> ()
      n21 = property on="dargestellte Größe 2" class="Ring (strict)"("AllowUndefVals"=w265) -> ()  [unwired: 2 in, 2 out]
      n22 = property on="Zeitachse2" class="Ring (strict)"("AllowUndefVals"=w265) -> ()  [unwired: 2 in, 2 out]
      n23 = property on="Zeitachse1" class="Ring (strict)"("AllowUndefVals"=w265) -> ()  [unwired: 2 in, 2 out]
      n24 = property on="dargestellte Größe 1" class="Ring (strict)"("AllowUndefVals"=w265) -> ()  [unwired: 2 in, 2 out]
      n25 = property on="Methode" class="Ring (strict)"("AllowUndefVals"=w265) -> ()  [unwired: 2 in, 2 out]
      n26 = local write "global stop RT"(w266) -> ()
      n27 = global write "gvbooleschRT.vi" "global stop RT"(w266) -> ()
      n28 = global write "GVZeitenZyklen.vi" "ZyklusNummern"(w162) -> ()
      n29 = global write "GVZeitenZyklen.vi" "ZyklusNummernGesamt"(w162) -> ()
      n30 = global write "GVZeitenZyklen.vi" "Big Ben, Methodenzeit, Zykluszeit0, Zykluszeit1, Zykluszeit2A, Zykluszeit2B"(w165) -> ()
      n31 = property on="Methode" class="Ring (strict)"("Value"=w145) -> ()  [unwired: 2 in, 2 out]
      n32 = Initialize Array(-1.0 ("Element"), 6 ("Dimension")) -> (w172:dbl[])
      n33 = Initialize Array(FALSE, 10 ("Dimension")) -> (w180:bool[])
      n34 = Initialize Array(-1.0 ("Element"), 96 ("Dimension")) -> (w173:dbl[])
      n35 = local write "LH-Gruppe"(w83) -> ()
      n36 = Strip Path(path=w63) -> (stripped path=w64:path)  [unwired: 1 out]
      n37 = Strip Path(path=w68) -> (stripped path=w65:path, name=w67:string)
      n38 = global write "GVZwangs.vi" "ZwangsFPGABoolesch!"(w180) -> ()
      n39 = global write "GVZwangs.vi" "ZwangsFPGABoolesch?"(w180) -> ()
      n40 = global write "GVTrapsMachs.vi" "Traps/Machs"(w172) -> ()
      n41 = global write "GVAIs.vi" "AIs"(w173) -> ()
      n42 = for {
        tunnel: w179 -> [w418] mode=indexing
        tunnel: [w415] -> w178 mode=indexing
        tunnel: [w413] -> w177 mode=indexing
        n43 = Initialize Array(0.0 ("Element"), w418) -> (w416:dbl[])
        n44 = Initialize Array(FALSE, w418) -> (w414:bool[])
        n45 = Bundle(w416) -> (w415:cluster{dbl[]})  [unwired: 1 in]
        n46 = Bundle(w414) -> (w413:cluster{bool[]})  [unwired: 1 in]
      }
      n47 = Bundle("DIOsMod0Name"=w125, "DIOsMod1Name"=w126, "DIOsMod2AName"=w124, "DIOsMod2BName"=w123, "ReglerNameMod0"=w138, "ReglerNameMod1"=w137, "ReglerNameMod2A"=w136, "ReglerNameMod2B"=w135, "LangsameHeizungen"=w206) -> (w268:T17)  [unwired: 1 in]
      n48 = Build Array (concatenate)(w138, w137, w136, w135) -> (w160:string[])
      n49 = Build Array (concatenate)(w228, w227, w226, w225) -> (w279:string[])
      n50 = Build Array (concatenate)(w232, w231, w230, w229) -> (w280:string[])
      n51 = Build Array (concatenate)(w224, w223, w222, w221) -> (w272:dbl[])
      n52 = Build Array (concatenate)(w220, w219, w218, w217) -> (w278:string[])
      n53 = Build Array (concatenate)(w138, w137, w136, w135) -> (→"HorstRegler":string[])
      n54 = Build Array (concatenate)(w95, w94, w93, w92) -> (w91:dbl[][])
      n55 = Array Size(array=w140) -> (size(s)=w75:i32)
      n56 = Build Array(w189, w188, w187, w186) -> (w185:i32[][])
      n57 = Array Size(array=w206) -> (size(s)=w205:i32)
      n58 = Add Array Elements(numeric array=w179) -> (sum=w264:i32)
      n59 = Array Size(array=w176) -> (size(s)=w175:i32)
      n60 = Index Array(array=w146, index=w145) -> (element=w144:T18)
      n61 = Add Array Elements(numeric array=w179) -> (sum=w191:i32)
      n62 = Decrement(x=w201) -> (x-1=w200:i32[])
      n63 = Build Cluster Array(w189, w188, w187, w186) -> (w271:cluster{"DIOsMod2BNr":i32[]}[])
      n64 = Build Array (concatenate)(w212, w211, w210) -> (w151:string[])
      n65 = Index Array(array=w213, index (col)=2 ("Deaktivierter Index (Spalte)")) -> (element=w260:dbl[])  [unwired: 1 in]
      n66 = Index Array(array=w213, index (col)=0 ("Deaktivierter Index (Spalte)")) -> (element=w258:dbl[])  [unwired: 1 in]
      n67 = Index Array(array=w213, index (col)=1 ("Deaktivierter Index (Spalte)")) -> (element=w259:dbl[])  [unwired: 1 in]
      n68 = Concatenate Strings("?SE0,SETP,0800" ("string"), "\r\n") -> (w102:string)
      n69 = Concatenate Strings("?SE0,SETP,2100" ("string"), "\r\n") -> (w109:string)
      n70 = Strip Path(path=w60) -> (stripped path=w59:path, name=w62:string)
      n71 = Concatenate Strings(w67, "Backup" ("string")) -> (w49:string)
      n72 = Build Path(base path=w64, name or relative path=w54) -> (appended path=w55:path)
      n73 = Build Path(base path=w65, name or relative path=w49) -> (appended path=w50:path)
      n74 = Concatenate Strings(w62, "Backup" ("string")) -> (w45:string)
      n75 = for {
        tunnel: w271 -> [w443] mode=indexing
        tunnel: [w444] -> w270 mode=indexing
        n76 = Unbundle(w443) -> ("DIOsMod2BNr"=w442:i32[])
        n77 = Array Size(array=w442) -> (size(s)=w444:i32)
      }
      n78 = property on="Methode" class="Ring (strict)"("Strings []"=w273) -> ()  [unwired: 2 in, 2 out]
      n79 = Bundle("Modul1/AI sicherer Bereich"=w100, "Modul2/AI sicherer Bereich"=w99, "Modul3/AI sicherer Bereich"=w98, "Traps/Machs sicherer Bereich"=w97, w91, "Metavariablen grüner Bereich"=w90) -> (w96:T19)  [unwired: 1 in]
      n80 = Build Array (concatenate)(w173, w172) -> (w171:dbl[])
      n81 = Initialize Array(FALSE, w75) -> (w72:bool[])
      n82 = Array Size(array=w185) -> (size(s)=w184:i32[])
      n83 = Unbundle(w144) -> ("SPMPV"=w143:i32[])  [unwired: 44 out]
      n84 = Open/Create/Replace File(file path (use dialog)=path "c:/fromcriordy.txt" ("Dateipfad (Dialog verwenden)"), operation (0:open)=T13."replace or create" ("Operation (0:Öffnen)")) -> (refnum out=w237:refnum<file>, error out=w238:errorcluster)  [unwired: 4 in, 1 out]
      n85 = Initialize Array(0.0 ("element"), w75) -> (w73:dbl[])
      n86 = Initialize Array(0.0 ("Element"), w191) -> (w190:dbl[])
      n87 = Build Path(base path=w59, name or relative path=w45) -> (appended path=w44:path)
      n88 = Get Date/Time In Seconds() -> (seconds since 1Jan1904=w133:timestamp)
      n89 = Initialize Array(FALSE, w175) -> (w170:bool[])
      n90 = Multiply(x=w200, y=32) -> (x*y=w203:i32[])
      n91 = Initialize Array(-1.0, w191) -> (w193:dbl[])
      n92 = Array Subset(array=w151, index=32 ("Index"), length=32 ("Länge")) -> (→"AIs2":string[])
      n93 = Array Subset(array=w151, index=0 ("Index"), length=32 ("Länge")) -> (→"AIs1":string[])
      n94 = Array Subset(array=w151, index=64 ("Index"), length=32 ("Länge")) -> (→"AIs3":string[])
      n95 = global write "GVHK1Hz.vi" "Mod1Mod2Mod3/AITrapsMachs1Hz"(w171) -> ()
      n96 = global write "GVMetavariablen.vi" "Metavariablen"(w73) -> ()
      n97 = global write "GVHeizenLH.vi" "Heizen?LH"(w170) -> ()
      n98 = global write "GVZwangs.vi" "ZwangsLangsameHeizungenAn!"(w170) -> ()
      n99 = for {
        tunnel: w184 -> [w423] mode=indexing
        tunnel: [w420] -> w183 mode=indexing
        n100 = Initialize Array(FALSE, w423) -> (w421:bool[])
        n101 = Bundle(w421) -> (w420:cluster{bool[]})  [unwired: 1 in]
      }
      n102 = global write "GVHorstSP.vi" "HorstSP"(w190) -> ()
      n103 = global write "GVZwangs.vi" "ZwangsLangsameHeizungenAn?"(w170) -> ()
      n104 = global write "GVMetavariablen.vi" "MVFixwert"(w73) -> ()
      n105 = Add(x=w203, y=w176) -> (x+y=w202:i32[])
      n106 = Close File(refnum=w237, error in=w238) -> (path=w269:path)  [unwired: 1 out]
      n107 = Format Date/Time String(time format string (%c)="%Y-%m-%d--%H-%M" ("Zeitformatierungs-String (%c)"), seconds (now)=w133) -> (date/time string=w46:string)  [unwired: 1 in]
      n108 = Concatenate Strings(w49, w46) -> (w51:string)
      n109 = Concatenate Strings(w45, w46) -> (w47:string)
      n110 = Build Path(base path=w50, name or relative path=w51) -> (appended path=w48:path)
      n111 = Build Path(base path=w44, name or relative path=w47) -> (appended path=w43:path)
      n112 = Concatenate Strings(w54, w46) -> (w53:string)
      n113 = Create Folder(path (use dialog)=w48) -> (created path=w57:path)  [unwired: 2 in, 2 out]
      n114 = Create Folder(path (use dialog)=w43) -> (created path=w56:path)  [unwired: 2 in, 2 out]
      n115 = Bundle("created path"=w57, "created path"=w56) -> (w58:T20)  [unwired: 1 in]
      n116 = String To Byte Array(string=w102) -> (unsigned byte array=w104:u8[])
      n117 = String To Byte Array(string=w109) -> (unsigned byte array=w114:u8[])
      n118 = global write "GVMetavariablen.vi" "MVFix?"(w72) -> ()
      n119 = Index Array(array=w143, index=0) -> (element=w141:i32)
      n120 = Build Path(base path=w55, name or relative path=w53) -> (appended path=w52:path)
      n121 = call "FPGA-Start-15-07-17.vi"() -> ("error out"=w88:errorcluster, "FPGA VI Reference Out"=w87:refnum<k20>)  [unwired: 2 in]
      n122 = local write "MVFix?"(w72) -> ()
      n123 = local write "MVFixwert"(w73) -> ()
      n124 = global write "GVMWHorst.vi" "MWHorst"(w193) -> ()
      n125 = global write "GVVentilposition.vi" "Ventilposition"(w141) -> ()
      n126 = Build Array (concatenate)(string[] ["Jahr", "Monat", "Tag", "Stunde", "Minute", "Sekunde"] ("Array"), string[] ["Datei Nr.", "Methode Nr.", "Zyklusnr. Mod0", "Zyklusnr. Mod1", "Zyklusnr. Mod2A", "Zyklusnr. Mod2B"], w275, w151, w76, w160, "Probenvolumen1", "Probenvolumen2", "Ventilposition" ("element"), string[] ["CPU Total", "CPU Time critical", "CPU Timed Structures", "CPU High", "CPU Above normal", "CPU Normal", "CPU Background", "CPU Idle", "CPU ISR", "Memory", "SekundenTotalBrutal"]) -> (w277:string[])
      n127 = Build Array (concatenate)(w76, w160) -> (w159:string[])
      n128 = Build Array (concatenate)(w151, w76, w160) -> (w158:string[])
      n129 = Join Numbers(hi=w104, lo=u8 5) -> ((hi.lo)=w101:u16[])
      n130 = Join Numbers(hi=w114, lo=u8 6) -> ((hi.lo)=w112:u16[])
      n131 = Split 1D Array(array=w275, index=2 ("Index")) -> (second subarray=w267:string[])  [unwired: 1 out]
      n132 = Concatenate Strings("HK " ("String"), w46) -> (w120:string)
      n133 = Concatenate Strings("ECD1 " ("String"), w46) -> (w118:string)
      n134 = Concatenate Strings("ECD2 " ("String"), w46) -> (w116:string)
      n135 = property on="dargestellte Größe 1" class="Ring (strict)"("Strings []"=w158) -> ()  [unwired: 2 in, 2 out]
      n136 = global write "GVZwangs.vi" "ZwangsHorst!"(w178) -> ()
      n137 = global write "GVZwangs.vi" "ZwangsHorst?"(w177) -> ()
      n138 = xnode "Invoke Method"("FPGA VI Reference In"=w87, "Data"=w101) -> ("FPGA VI Reference Out"=w107:refnum<k20>)  [unwired: 2 in, 2 out]
      n139 = property on="dargestellte Größe 2" class="Ring (strict)"("Strings []"=w158) -> ()  [unwired: 2 in, 2 out]
      n140 = property on="dargestellte Größe 3" class="Ring (strict)"("Strings []"=w159) -> ()  [unwired: 2 in, 2 out]
      n141 = property on="Zeitachse2" class="Ring (strict)"("Strings []"=w267) -> ()  [unwired: 2 in, 2 out]
      n142 = property on="Zeitachse1" class="Ring (strict)"("Strings []"=w267) -> ()  [unwired: 2 in, 2 out]
      n143 = xnode "Invoke Method"("FPGA VI Reference In"=w107, "Data"=w112) -> ("FPGA VI Reference Out"=w86:refnum<k20>)  [unwired: 2 in, 2 out]
      n144 = Create Folder(path (use dialog)=w52) -> (created path=w69:path)  [unwired: 2 in, 2 out]
      n145 = Build Path(base path=w63, name or relative path=w120) -> (appended path=w78:path)
      n146 = Build Path(base path=w68, name or relative path=w118) -> (appended path=w130:path)
      n147 = Build Path(base path=w60, name or relative path=w116) -> (appended path=w132:path)
      n148 = Strip Path(path=w81) -> (name=w80:string)  [unwired: 1 out]
      n149 = global write "GVZwangs.vi" "ZwangsDIO!"(w183) -> ()
      n150 = global write "GVZwangs.vi" "ZwangsDIO?"(w183) -> ()
      n151 = call "MPVSenden-15-07-17.vi"("Ventilposition"=0, "FPGA VI Reference In"=w86) -> ("FPGA VI Reference Out"=w84:refnum<k20>)  [unwired: 1 in, 2 out]
      n152 = Build Path(base path=w69, name or relative path=w80) -> (appended path=w71:path)
      n153 = Create Folder(path (use dialog)=w78) -> (created path=w82:path)  [unwired: 2 in, 2 out]
      n154 = Create Folder(path (use dialog)=w130) -> (created path=w129:path)  [unwired: 2 in, 2 out]
      n155 = Create Folder(path (use dialog)=w132) -> (created path=w131:path)  [unwired: 2 in, 2 out]
      n156 = Copy(10:w71, 11:w81) -> ()  [unwired: 3 in, 3 out]
      n157 = Strip Path(path=w77) -> (name=w79:string)  [unwired: 1 out]
      n158 = case shown="True" w147 {
        tunnel: [w434 w439] -> w251
        tunnel: [w434 w438] -> w250
        tunnel: w82 -> [_ w437]
        tunnel: w209 -> [_ w436]
        tunnel: w145 -> [_ w435]
        frame False {
          w434 = refnum<k34> refnum ("tdms1")
        }
        frame True {
          n159 = call "TDMS0.vi"("Startmethode"=w435, "Dateiname"=w436, "Dateiordner"=w437) -> ("tdms1"=w438:refnum<k34>, "tdms0"=w439:refnum<k34>)
          n160 = global write "GVaktuelleTDMS.vi" "aktuelleTDMS-DateiHK"(w439) -> ()
        }
      }
      n161 = case shown="True" w147 {
        tunnel: [w424 w433] -> w249
        tunnel: [w424 w432] -> w248
        tunnel: [w424 w431] -> w247
        tunnel: [w424 w430] -> w246
        tunnel: w129 -> [_ w429]
        tunnel: w208 -> [_ w428]
        tunnel: w131 -> [_ w427]
        tunnel: w207 -> [_ w426]
        tunnel: w145 -> [_ w425]
        frame False {
          w424 = refnum<k34> refnum ("tdms0")
        }
        frame True {
          n162 = call "TDMS0.vi"("Startmethode"=w425, "Dateiname"=w428, "Dateiordner"=w429) -> ("tdms1"=w432:refnum<k34>, "tdms0"=w433:refnum<k34>)
          n163 = call "TDMS0.vi"("Startmethode"=w425, "Dateiname"=w426, "Dateiordner"=w427) -> ("tdms1"=w430:refnum<k34>, "tdms0"=w431:refnum<k34>)
          n164 = global write "GVaktuelleTDMS.vi" "aktuelleTDMS-DateiECD1"(w433) -> ()
          n165 = global write "GVaktuelleTDMS.vi" "aktuelleTDMS-DateiECD2"(w431) -> ()
        }
      }
      n166 = Build Path(base path=w69, name or relative path=w79) -> (appended path=w70:path)
      n167 = Copy(10:w70, 11:w77) -> ()  [unwired: 3 in, 3 out]
      n168 = Open/Create/Replace File(file path (use dialog)=path "c:/fromcriocmd.txt" ("Pfad MS-Datei CRIO"), operation (0:open)=T13."replace or create" ("Operation (0:Öffnen)")) -> (refnum out=w243:refnum<file>, error out=w242:errorcluster)  [unwired: 4 in, 1 out]
      n169 = Write to Text File(file (use dialog)=w243, text="time=yyyymmddhhmmss\ncycle=005\ninfo=1234567890123456789012345678901234567890123456789012345678901234567890123456789012345678901234567890\nlength=100\ncmd=cycle" ("Text0 MS-Datei"), error in=w242) -> (refnum out=w240:refnum<file>, error out=w239:errorcluster)  [unwired: 1 in, 1 out]
      n170 = Bundle("created path"=w82, "created path"=w129, "created path"=w131, "Dateiname Housekeeping"=w209, "DateinameECD1"=w208, "DateinameECD2"=w207, "tdms0"=w251, "tdms1"=w250, "tdms0"=w249, "tdms1"=w248, "tdms0"=w247, "tdms1"=w246) -> (w252:T21)  [unwired: 1 in]
      n171 = call "AIKoeffSortieren.vi"("Modul3/AI koeff"=w214, "Modul2/AI koeff"=w215, "Modul1/AI koeff"=w216) -> ("P0"=w255:dbl[], "P1"=w256:dbl[], "P2"=w257:dbl[])
      n172 = Close File(refnum=w240, error in=w239) -> (path=w234:path)  [unwired: 1 out]
      "schnelle Heizungen" <- w76
    }
    frame #1 {
      w454 = dbl[] [-1.0]
      w525 = 0
      w500 = 0 ("Zyklusnummer1")
      n173 = Add Array Elements(numeric array=w474) -> (sum=w473:i32)
      n174 = Array Size(array=w482) -> (size(s)=w503:i32)
      n175 = Unbundle(w499) -> ("created path"=w498:path, "created path"=w496:path, "created path"=w495:path, "Dateiname Housekeeping"=w497:string, "DateinameECD1"=w494:string, "DateinameECD2"=w493:string, "tdms0"=w492:refnum<k34>, "tdms1"=w491:refnum<k34>, "tdms0"=w490:refnum<k34>, "tdms1"=w489:refnum<k34>, "tdms0"=w488:refnum<k34>, "tdms1"=w487:refnum<k34>)
      n176 = Index Array(array=w475, index #1=0 ("Index"), index #2=1 ("Index"), index #3=2 ("Index"), index #4=3 ("Index")) -> (element #1=w514:i32, element #2=w513:i32, element #3=w516:i32, element #4=w515:i32)
      n177 = flat-sequence {
        frame #0 {
          n178 = global write "Emulate Licor output GV.vi" "Emulator an?"(FALSE ("Emulator an?")) -> ()
        }
        frame #1 {
          n179 = control-ref of="GUI_Cluster_sdv"() -> (w553:refnum<vi>)
          n180 = control-ref of="GUI_Cluster_Graph"() -> (w555:refnum<vi>)
          n181 = control-ref of="GUI_Cluster_Parameter"() -> (w554:refnum<vi>)
          n182 = call "licore (main).vi"("GUI_Cluster_Graph (extern)"=w555, "GUI_Cluster_Parameter (extern)"=w554, "GUI_Cluster_sdv (extern)"=w553) -> ()  [unwired: 13 in]
        }
      }
      n183 = while {
        shift-right: ["Methode"] -> _
        shift-left: w551 -> [w1474]
        stop <- w1476 stop-if-true
        n184 = call "Bis zum nächsten Vielfachen warten7"("Count(mSec)"=u32 1000) -> ()  [unwired: 1 out]
        n185 = Not Equal?(x=w1474, y="Methode") -> (x != y?=w1472:bool)
        n186 = global read "gvbooleschRT.vi" "global stop RT"() -> (w1476:bool)
        n187 = global write "GVMethodenwechsel.vi" "Methodenwechsel?"(w1472) -> ()
      }
      n188 = call <vilib>:"Space Constant.vi"() -> ("String"=w460:string)
      n189 = while {
        tunnel: w478 -> [w921]
        tunnel: w547 -> [w924]
        tunnel: w546 -> [w923]
        tunnel: w545 -> [w922]
        shift-right: [w926] -> _
        shift-left: errorcluster {"status"=FALSE, "code"=0, "source"=""} ("error out") -> [w925]
        stop <- w927 stop-if-true
        n190 = call "AIsFIFORT-15-07-17.vi"("FPGA VI Reference In"=w921, "P2"=w924, "P1"=w923, "P0"=w922, "error in"=w925) -> ("error out"=w926:errorcluster)
        "AIsFIFOread" <- w926
        n191 = global read "gvbooleschRT.vi" "global stop RT"() -> (w927:bool)
      }
      n192 = while {
        tunnel: w478 -> [w928]
        tunnel: w453 -> [w931]
        tunnel: w452 -> [w930]
        tunnel: w451 -> [w929]
        shift-right: [w933] -> _
        shift-left: errorcluster {"status"=FALSE, "code"=0, "source"=""} ("error out") -> [w932]
        stop <- w935 stop-if-true
        n193 = call "Bis zum nächsten Vielfachen warten16"("Count(mSec)"=u32 100) -> ()  [unwired: 1 out]
        n194 = call "TrapsMachMitteln-15-07-17.vi"("FPGA VI Reference In"=w928, "Traps/MachKoeff2"=w931, "Traps/MachKoeff1"=w930, "Traps/MachKoeff0"=w929, "error in"=w932) -> ("error out"=w933:errorcluster)
        "MWTrapsMachs" <- w933
        n195 = global read "gvbooleschRT.vi" "global stop RT"() -> (w935:bool)
      }
      n196 = for {
        N: 1 -> [_]
        tunnel: w478 -> [w936]
        tunnel: [w936] -> w505
        n197 = call "Warten8"("Count(mSec)"=u32 100) -> ()  [unwired: 1 out]
      }
      n198 = Build Array(w460) -> (w459:string[])
      n199 = Initialize Array(-1 ("Element"), 4 ("Dimension")) -> (w476:i32[])
      n200 = global read "GVVentilposition.vi" "Ventilposition"() -> (w484:i32)
      n201 = Add(x=w516, y=w515) -> (x+y=w512:i32)
      n202 = Bundle(w459, w459, w459) -> (w523:cluster{string[], string[], string[]})  [unwired: 1 in]
      n203 = Index Array(array=w469, index=w467) -> (element=w468:T18)
      n204 = Initialize Array(cluster{"output high":dbl, "output low":dbl} {"output high"=99999.0, "output low"=0.0} ("output range"), w503) -> (w483:cluster{"output high":dbl, "output low":dbl}[])
      n205 = while {
        tunnel: w550 -> [w1052]
        shift-right: [w1051] -> _
        shift-left: w469 -> [w1033]
        tunnel: w483 -> [w1050]
        tunnel: w482 -> [w1049]
        tunnel: w478 -> [w1048]
        tunnel: w481 -> [w1047]
        tunnel: w480 -> [w1046]
        shift-right: [w1040] -> _
        shift-left: 0 -> [w1045]
        tunnel: w478 -> [w1044]
        tunnel: w477 -> [w1043]
        shift-right: [w1039] -> _
        shift-left: w476 -> [w1042]
        tunnel: w475 -> [w1034]
        tunnel: w474 -> [w1035]
        tunnel: w473 -> [w1036]
        tunnel: w472 -> [w1037]
        tunnel: w471 -> [w1038]
        tunnel: w470 -> [w1041]
        shift-right: [w957] -> _
        shift-left: w468 -> [w956]
        tunnel: w453 -> [w942]
        tunnel: w452 -> [w943]
        tunnel: w451 -> [w944]
        tunnel: w446 -> [w945]
        tunnel: w445 -> [w941]
        i -> [w960]
        stop <- w1053 stop-if-true
        w950 = 0  # ZeileMainMach2
        w951 = 0  # ZeileMainMach1
        w1001 = FALSE
        w1000 = 0.0
        w1002 = 0  # ZeilennummerMPV
        w1006 = cluster{dbl[], dbl[]} {[], []}
        w1015 = dbl[] []
        w1019 = 0  # ZeilePreMach2
        w1020 = 0  # ZeilePreMach1
        w1021 = 0  # ZeileFPGAFixp
        w1022 = 0  # ZeileFPGAPID
        w1023 = 0  # ZeileFPGABoolesch
        w1024 = i32[] [0, 0, 0, 0]  # ZeilennummernHorst
        w1025 = i32[] [0, 0, 0, 0]  # ZeilennummernDIOs
        n206 = Unbundle(w941) -> ("created path"=w940:path, "created path"=w939:path)
        n207 = Unbundle(w956) -> ("Zykluslängen [s]"=w938:dbl[], "ZeitpktDIOsMod0"=w999:dbl[], "ZeitpktDIOsMod1"=w998:dbl[], "ZeitpktDIOsMod2A"=w997:dbl[], "ZeitpktDIOsMod2B"=w996:dbl[], "DIOsSPMod0"=w995:bool[][], "DIOsSPMod1"=w994:bool[][], "DIOsSPMod2A"=w993:bool[][], "DIOsSPMod2B"=w992:bool[][], "Mod0HorstZeitpkt"=w991:dbl[], "Mod1HorstZeitpkt"=w990:dbl[], "Mod2AHorstZeitpkt"=w989:dbl[], "Mod2BHorstZeitpkt"=w988:dbl[], "HorstSPMod0"=w987:dbl[][], "HorstSPMod1"=w986:dbl[][], "HorstSPMod2A"=w985:dbl[][], "HorstSPMod2B"=w984:dbl[][], "LHSetpoints"=w983:dbl[], "LHHeizen?"=w982:bool[], "ZPktFPGABoolesch"=w981:dbl[], "FPGABoolesch"=w980:bool[][], "ZeitpktFPGAPID"=w979:dbl[], "FPGAPID"=w978:T22, "ZeitpktFPGAFixp"=w977:dbl[], w976:dbl[][], "t_PreMach1"=w975:dbl[], "T_PreMach1"=w974:dbl[], "t_PreMach2"=w973:dbl[], "T_PreMach2"=w972:dbl[], "PIDs für \"träge\" Heizungen"=w971:T23, "Zwangsbedingungen"=w970:dbl[][], "Dateien fürs MS schicken?"=w969:bool, "ZeitpunkteMPV"=w968:dbl[], "SPMPV"=w967:i32[], "ZeitpktMS-1"=w966:dbl, "ZeitpktMS-2"=w965:dbl, "Int.Start1"=w964:dbl, "Int.Stop1"=w963:dbl, "Int.Start2"=w962:dbl, "Int.Stop2"=w961:dbl, "t_MainMach1"=w955:dbl[], "T_MainMach1"=w954:dbl[], "t_MainMach2"=w953:dbl[], "T_MainMach2"=w952:dbl[])  [unwired: 1 out]
        n208 = while {
          tunnel: w938 -> [w1086]
          tunnel: w939 -> [w1076]
          stop <- w1075 stop-if-true
          n209 = global read "GVZeitenZyklen.vi" "Big Ben, Methodenzeit, Zykluszeit0, Zykluszeit1, Zykluszeit2A, Zykluszeit2B"() -> (w1084:dbl[])
          n210 = Index Array(array=w1084, index=5) -> (element=w1082:dbl)
          n211 = global read "GVZeitenZyklen.vi" "ZyklusNummernGesamt"() -> (w1087:i32[])
          n212 = call "Wait Until Next Multiple2"("Count(mSec)"=u32 100) -> ()  [unwired: 1 out]
          n213 = Index Array(array=w1086, index=3) -> (element=w1081:dbl)
          n214 = Subtract(x=w1081, y=0.2) -> (x-y=w1079:dbl)
          n215 = Greater Or Equal?(x=w1082, y=w1079) -> (x >= y?=w1078:bool)
          n216 = global read "GVChroms.vi" "ECD2Chrom"() -> (w1077:dbl[])
          n217 = case shown="True" w1078 {
            tunnel: w1087 -> [_ w1095]
            tunnel: w1077 -> [_ w1094]
            tunnel: w1076 -> [_ w1093]
            frame False {
            }
            frame True {
              n218 = flat-sequence {
                tunnel: w1095 -> [w1111]
                tunnel: w1094 -> [w1098]
                tunnel: w1093 -> [w1097]
                frame #0 {
                  n219 = Index Array(array=w1111, index=3) -> (element=w1109:i32)
                  n220 = Number To Decimal String(number=w1109, width (-)=i16 4) -> (decimal integer string=w1107:string)
                  n221 = Concatenate Strings(w1107, "ECD2.hag" ("string")) -> (w1105:string)
                  n222 = Build Path(base path=w1097, name or relative path=w1105) -> (appended path=w1096:path)
                  n223 = Open/Create/Replace File(file path (use dialog)=w1096, operation (0:open)=T13."replace or create") -> (refnum out=w1104:refnum<file>, error out=w1103:errorcluster)  [unwired: 4 in, 1 out]
                  n224 = Write to Binary File(file (use dialog)=w1104, data=w1098, error in=w1103) -> (refnum out=w1102:refnum<file>, error out=w1101:errorcluster)  [unwired: 3 in, 1 out]
                  n225 = Close File(refnum=w1102, error in=w1101) -> (error out=→"ECD2dataBackup":errorcluster)  [unwired: 1 out]
                }
                frame #1 {
                  n226 = call "Wait2"("Count(mSec)"=u32 2000) -> ()  [unwired: 1 out]
                }
              }
            }
          }
          n227 = global read "GVMethodenwechsel.vi" "Methodenwechsel?"() -> (w1090:bool)
          n228 = global read "gvbooleschRT.vi" "global stop RT"() -> (w1091:bool)
          n229 = Or(x=w1090, y=w1091) -> (x .or. y?=w1092:bool)
          n230 = local read "veränderte Methode benutzen"() -> (w1089:bool)
          n231 = Or(x=w1092, y=w1089) -> (x .or. y?=w1075:bool)
        }
        n232 = while {
          tunnel: w938 -> [w1123]
          tunnel: w940 -> [w1113]
          stop <- w1127 stop-if-true
          n233 = global read "GVZeitenZyklen.vi" "Big Ben, Methodenzeit, Zykluszeit0, Zykluszeit1, Zykluszeit2A, Zykluszeit2B"() -> (w1121:dbl[])
          n234 = Index Array(array=w1121, index=4) -> (element=w1119:dbl)
          n235 = global read "GVZeitenZyklen.vi" "ZyklusNummernGesamt"() -> (w1124:i32[])
          n236 = call "Wait Until Next Multiple"("Count(mSec)"=u32 100) -> ()  [unwired: 1 out]
          n237 = Index Array(array=w1123, index=2) -> (element=w1118:dbl)
          n238 = Subtract(x=w1118, y=0.2) -> (x-y=w1116:dbl)
          n239 = Greater Or Equal?(x=w1119, y=w1116) -> (x >= y?=w1115:bool)
          n240 = global read "GVChroms.vi" "ECD1Chrom"() -> (w1114:dbl[])
          n241 = case shown="True" w1115 {
            tunnel: w1124 -> [_ w1133]
            tunnel: w1114 -> [_ w1132]
            tunnel: w1113 -> [_ w1131]
            frame False {
            }
            frame True {
              n242 = flat-sequence {
                tunnel: w1133 -> [w1149]
                tunnel: w1132 -> [w1136]
                tunnel: w1131 -> [w1135]
                frame #0 {
                  n243 = Index Array(array=w1149, index=2) -> (element=w1147:i32)
                  n244 = Number To Decimal String(number=w1147, width (-)=i16 4) -> (decimal integer string=w1145:string)
                  n245 = Concatenate Strings(w1145, "ECD1.hag" ("string")) -> (w1143:string)
                  n246 = Build Path(base path=w1135, name or relative path=w1143) -> (appended path=w1134:path)
                  n247 = Open/Create/Replace File(file path (use dialog)=w1134, operation (0:open)=T13."replace or create") -> (refnum out=w1142:refnum<file>, error out=w1141:errorcluster)  [unwired: 4 in, 1 out]
                  n248 = Write to Binary File(file (use dialog)=w1142, data=w1136, error in=w1141) -> (refnum out=w1140:refnum<file>, error out=w1139:errorcluster)  [unwired: 3 in, 1 out]
                  n249 = Close File(refnum=w1140, error in=w1139) -> (error out=→"ECD1dataBackup":errorcluster)  [unwired: 1 out]
                }
                frame #1 {
                  n250 = call "Wait"("Count(mSec)"=u32 2000) -> ()  [unwired: 1 out]
                }
              }
            }
          }
          n251 = global read "GVMethodenwechsel.vi" "Methodenwechsel?"() -> (w1128:bool)
          n252 = global read "gvbooleschRT.vi" "global stop RT"() -> (w1129:bool)
          n253 = Or(x=w1128, y=w1129) -> (x .or. y?=w1130:bool)
          n254 = local read "veränderte Methode benutzen"() -> (w1126:bool)
          n255 = Or(x=w1130, y=w1126) -> (x .or. y?=w1127:bool)
        }
        n256 = Add(x=w1042, y=1) -> (x+y=w1010:i32[])
        n257 = local read "Methode"() -> (w959:i32)
        n258 = Build Cluster Array(w995, w994, w993, w992) -> (w1029:cluster{"DIOsSPMod2B":bool[][]}[])
        n259 = Build Cluster Array(w987, w986, w985, w984) -> (w1027:cluster{"HorstSPMod2B":dbl[][]}[])
        n260 = Build Cluster Array(w999, w998, w997, w996) -> (w1030:cluster{"ZeitpktDIOsMod2B":dbl[]}[])
        n261 = Build Cluster Array(w991, w990, w989, w988) -> (w1028:cluster{"Mod2BHorstZeitpkt":dbl[]}[])
        n262 = Equal?(x=w960, y=0) -> (x = y?=w1031:bool)
        n263 = while {
          tunnel: w938 -> [w1061]
          stop <- w1064 stop-if-true
          n264 = global read "GVZeitenZyklen.vi" "Big Ben, Methodenzeit, Zykluszeit0, Zykluszeit1, Zykluszeit2A, Zykluszeit2B"() -> (w1070:dbl[])
          n265 = To Long Integer(number="Zyklus") -> (32bit integer=w1056:i32)
          n266 = Index Array(array=w1061, index=w1056) -> (element=w1060:dbl)
          n267 = Subtract(x=w1060, y=1.0) -> (x-y=w1058:dbl)
          n268 = Add(x=w1056, y=2) -> (x+y=w1054:i32)
          n269 = call "Wait3"("Count(mSec)"=u32 100) -> ()  [unwired: 1 out]
          n270 = global read "GVMethodenwechsel.vi" "Methodenwechsel?"() -> (w1066:bool)
          n271 = global read "gvbooleschRT.vi" "global stop RT"() -> (w1067:bool)
          n272 = local read "am Ende benutzen"() -> (w1069:bool)
          n273 = local read "veränderte Methode benutzen"() -> (w1062:bool)
          n274 = Index Array(array=w1070, index=w1054) -> (element=w1071:dbl)
          n275 = Or(x=w1066, y=w1067) -> (x .or. y?=w1065:bool)
          n276 = Greater Or Equal?(x=w1071, y=w1058) -> (x >= y?=w1072:bool)
          n277 = And(x=w1072, y=w1069) -> (x .and. y?=w1063:bool)
          n278 = case shown="True" w1063 {
            frame False {
            }
            frame True {
              n279 = local write "veränderte Methode benutzen"(TRUE ("veränderte Methode benutzen")) -> ()
              n280 = local write "am Ende benutzen"(FALSE ("am Ende benutzen")) -> ()
            }
          }
          n281 = Or(x=w1065, y=w1062) -> (x .or. y?=w1064:bool)
        }
        n282 = while {
          tunnel: w1035 -> [w1219]
          tunnel: w1038 -> [w1212]
          tunnel: w1037 -> [w1213]
          tunnel: w1034 -> [w1218]
          tunnel: w1036 -> [w1214]
          tunnel: w970 -> [w1215]
          stop <- w1221 stop-if-true
          n283 = call "Bis zum nächsten Vielfachen warten10"("Count(mSec)"=u32 1000) -> ()  [unwired: 1 out]
          n284 = local read "Methode"() -> (w1217:i32)
          n285 = global read "GVMethodenwechsel.vi" "Methodenwechsel?"() -> (w1223:bool)
          n286 = global read "gvbooleschRT.vi" "global stop RT"() -> (w1224:bool)
          n287 = case shown="True" "global stop RT" {
            frame False {
            }
            frame True {
              n288 = global write "gvbooleschRT.vi" "global stop RT"(TRUE ("global stop RT")) -> ()
            }
          }
          n289 = call "ZwangsbedingungenGV-15-07-17.vi"("AnzahlHorst"=w1212, "AnzahlHorst/Modul"=w1218, "AnzahlLH"=w1213, "AnzahlDIOs/Modul"=w1219, "AnzahlDIOs"=w1214, "Zwangsbedingungen"=w1215, "Methodennummer"=w1217) -> ("Methodennummer"=w1216:i32)  [unwired: 4 in]
          n290 = local write "Methode"(w1216) -> ()
          n291 = local read "veränderte Methode benutzen"() -> (w1222:bool)
          n292 = Compound Arithmetic op=OR(w1224, w1223, w1222) -> (w1221:bool)
        }
        n293 = global read "GVZeitenZyklen.vi" "ZyklusNummern"() -> (w1009:i32[])
        n294 = global read "GVZwangs.vi" "ZwangsHorst?"() -> (w1014:cluster{bool[]}[])
        n295 = global read "gvbooleschRT.vi" "global stop RT"() -> (w1053:bool)
        n296 = global read "GVZwangsMPV.vi" "ZwangsMPV?"() -> (w948:bool)
        n297 = global read "GVZwangs.vi" "ZwangsDIO?"() -> (w1013:cluster{bool[]}[])
        n298 = global read "GVaktuelleTDMS.vi" "aktuelleTDMS-DateiECD1"() -> (w1008:refnum<k34>)
        n299 = Bundle(w1030, w1029, w1028, w1027, "LHHeizen?"=w982, "ZPktFPGABoolesch"=w981, "FPGABoolesch"=w980, "ZeitpktFPGAPID"=w979, "FPGAPID"=w978, "ZeitpktFPGAFixp"=w977, w976, "t_PreMach1"=w975, "T_PreMach1"=w974, "t_PreMach2"=w973, "T_PreMach2"=w972, "ZeitpunkteMPV"=w968, "SPMPV"=w967, "t_MainMach1"=w955, "T_MainMach1"=w954, "t_MainMach2"=w953, "T_MainMach2"=w952) -> (w1026:T24)  [unwired: 1 in]
        n300 = Index Array(array=w1033, index=w959) -> (element=w958:T18)
        n301 = global read "GVZwangs.vi" "ZwangsFPGABoolesch?"() -> (w1012:bool[])
        n302 = while {
          tunnel: w1049 -> [w1202]
          tunnel: w1050 -> [w1205]
          tunnel: w1048 -> [w1206]
          tunnel: w983 -> [w1203]
          tunnel: w971 -> [w1204]
          shift-right: [w1200] -> _
          shift-left: errorcluster {"status"=FALSE, "code"=0, "source"=""} ("error out") -> [w1201]
          stop <- w1207 stop-if-true
          n303 = call "LH-15-07-17.vi"("FPGA VI Reference In"=w1206, "OutputRange"=w1205, "LHSetpoints"=w1203, "AIsLH"=w1202, "error in"=w1201, "LH-Gruppe"="LH-Gruppe", "PIDs für \"träge\" Heizungen"=w1204) -> ("error out"=w1200:errorcluster)
          "LH" <- w1200
          n304 = call "Bis zum nächsten Vielfachen warten12"("Count(mSec)"=u32 100) -> ()  [unwired: 1 out]
          n305 = global read "GVMethodenwechsel.vi" "Methodenwechsel?"() -> (w1209:bool)
          n306 = global read "gvbooleschRT.vi" "global stop RT"() -> (w1210:bool)
          n307 = local read "veränderte Methode benutzen"() -> (w1208:bool)
          n308 = Compound Arithmetic op=OR(w1210, w1209, w1208) -> (w1207:bool)
        }
        n309 = while {
          shift-right: [w1163] -> _
          shift-left: w1001 -> [w1167]
          shift-right: [w1162] -> _
          shift-left: w1000 -> [w1166]
          shift-right: [w1161] -> _
          shift-left: w1001 -> [w1165]
          shift-right: [w1160] -> _
          shift-left: w1000 -> [w1164]
          tunnel: w1041 -> [w1159]
          tunnel: w964 -> [w1154]
          tunnel: w963 -> [w1153]
          tunnel: w962 -> [w1152]
          tunnel: w961 -> [w1151]
          stop <- w1156 stop-if-true
          n310 = call "Integrieren.vi"("Integrieren1"=w1167, "Integral1"=w1166, "Integrieren2"=w1165, "Integral2"=w1164, "Int.Start1"=w1154, "Int.Stop1"=w1153, "Int.Start2"=w1152, "HorstProbenflußNr."=w1159, "Int.Stop2"=w1151) -> ("Integrieren1"=w1163:bool, "Integral1"=w1162:dbl, "Integrieren2"=w1161:bool, "Integral2"=w1160:dbl)  [unwired: 7 in]
          n311 = call "Bis zum nächsten Vielfachen warten9"("Count(mSec)"=u32 100) -> ()  [unwired: 1 out]
          n312 = global read "GVMethodenwechsel.vi" "Methodenwechsel?"() -> (w1157:bool)
          n313 = global read "gvbooleschRT.vi" "global stop RT"() -> (w1158:bool)
          n314 = local read "veränderte Methode benutzen"() -> (w1155:bool)
          n315 = Compound Arithmetic op=OR(w1158, w1157, w1155) -> (w1156:bool)
        }
        n316 = while "Zeit" {
          tunnel: w1031 -> [w1411]
          tunnel: w938 -> [w1409]
          tunnel: w1010 -> [w1404]
          tunnel: [w1403] -> w1039
          shift-right: [w1400] -> _
          shift-left: 0.0 -> [w1401]
          i -> [w1413]
          stop <- w1406 stop-if-true
          n317 = Equal?(x=w1413, y=0) -> (x = y?=w1402:bool)
          n318 = call "Bis zum nächsten Vielfachen warten15"("Count(mSec)"=u32 50) -> ()  [unwired: 1 out]
          n319 = call "BigBen-01-16.vi"("MethodenStartzeit"=w1401, "Methodenstart?"=w1402, "Programmstart?"=w1411, "Zykluslängen [s]"=w1409, "MethodenStartZyklusNummern"=w1404) -> ("MethodenStartzeit"=w1400:dbl, "ZyklusNummernGesamt"=w1403:i32[])  [unwired: 2 in]
          n320 = global read "GVMethodenwechsel.vi" "Methodenwechsel?"() -> (w1405:bool)
          n321 = global read "gvbooleschRT.vi" "global stop RT"() -> (w1410:bool)
          n322 = Or(x=w1405, y=w1410) -> (x .or. y?=w1407:bool)
          n323 = local read "veränderte Methode benutzen"() -> (w1408:bool)
          n324 = Or(x=w1408, y=w1407) -> (x .or. y?=w1406:bool)
        }
        n325 = Bundle(w1015, w1015, w1015, w1015) -> (w1016:cluster{dbl[], dbl[], dbl[], dbl[]})  [unwired: 1 in]
        n326 = while {
          tunnel: w1052 -> [w1426]
          shift-right: [w1417] -> _
          shift-left: w958 -> [w1425]
          tunnel: w959 -> [w1423]
          shift-right: [w1415] -> w1051
          shift-left: w1033 -> [w1424]
          tunnel: [w1416] -> w957
          stop <- w1419 stop-if-true
          n327 = call "Bis zum nächsten Vielfachen warten8"("Count(mSec)"=u32 500) -> ()  [unwired: 1 out]
          n328 = global read "GVMethodenwechsel.vi" "Methodenwechsel?"() -> (w1421:bool)
          n329 = global read "gvbooleschRT.vi" "global stop RT"() -> (w1420:bool)
          n330 = case shown="True" "Methode verändern" {
            tunnel: w1426 -> [_ w1448]
            tunnel: w1425 -> [w1445 w1447]
            tunnel: [w1445 w1446] -> w1417
            frame False {
            }
            frame True {
              n331 = call "methodeändern-15-07-17.vi"("->Methode"=w1447, "Namen"=w1448) -> ("Methode->"=w1446:T25)  [unwired: 1 in]
              n332 = property on="Methode verändern" class="Bool (strict)"("Value"=FALSE ("Methode verändern")) -> ()  [unwired: 2 in, 2 out]
            }
          }
          n333 = Compound Arithmetic op=OR(w1421, w1420, "veränderte Methode benutzen") -> (w1419:bool)
          n334 = case shown="True" "Methode speichern" {
            tunnel: w1417 -> [_ w1442]
            tunnel: w1424 -> [w1435 w1444]
            tunnel: w1423 -> [_ w1443]
            tunnel: [w1435 w1437] -> w1415
            frame False {
            }
            frame True {
              n335 = Replace Array Subset(array=w1444, new element=w1442, index=w1443) -> (w1437:T11)
              n336 = property on="Methode speichern" class="Bool (strict)"("Value"=FALSE ("Methode speichern")) -> ()  [unwired: 2 in, 2 out]
              n337 = Open/Create/Replace File(file path (use dialog)=path "c:/methoden.pery" ("Dateipfad (Dialog verwenden)"), operation (0:open)=T13."replace" ("Operation (0:Öffnen)")) -> (refnum out=w1439:refnum<file>)  [unwired: 4 in, 2 out]
              n338 = Write to Binary File(file (use dialog)=w1439, data=w1437) -> (refnum out=w1436:refnum<file>)  [unwired: 4 in, 2 out]
              n339 = Close File(refnum=w1436) -> ()  [unwired: 1 in, 2 out]
            }
          }
          n340 = case shown="True" "veränderte Methode benutzen" {
            tunnel: w1417 -> [_ w1432]
            tunnel: [w1429 w1432] -> w1416
            tunnel: w1415 -> [w1431 _]
            frame False {
              n341 = local read "Methode"() -> (w1430:i32)
              n342 = Index Array(array=w1431, index=w1430) -> (element=w1429:T18)
            }
            frame True {
              n343 = flat-sequence {
                frame #0 {
                  n344 = call "Warten"("Count(mSec)"=u32 1100) -> ()  [unwired: 1 out]
                }
                frame #1 {
                  n345 = property on="veränderte Methode benutzen" class="Bool (strict)"("Value"=FALSE ("Methode verändern")) -> ()  [unwired: 2 in, 2 out]
                }
              }
            }
          }
        }
        n346 = Bundle("ZyklusNummern"=w1009, "ZeilennummernDIOs"=w1025, "ZwangsDIO?"=w1013, "ZeilennummernHorst"=w1024, "ZwangsHorst?"=w1014, "ZeileFPGABoolesch"=w1023, "ZwangsFPGABoolesch?"=w1012, "ZeileFPGAPID"=w1022, "ZeileFPGAFixp"=w1021, "ZeilePreMach1"=w1020, "ZeilePreMach2"=w1019, "ZeilennummerMPV"=w1002, "ZeileMainMach1"=w951, "ZeileMainMach2"=w950, "ZwangsMPV?"=w948) -> (w1018:T26)  [unwired: 1 in]
        n347 = while {
          shift-right: [w1343] -> _
          shift-left: w1016 -> [w1350]
          shift-right: [w1342] -> _
          shift-left: w1016 -> [w1349]
          shift-right: [w1340] -> _
          shift-left: T16 {"Zyklus1"=0, "Zeitachse1"=0, "dargestellte Größe 1"=0, "Zyklus2"=0, "Zeitachse2"=0, "dargestellte Größe 2"=0} ("AnzeigeEinstellungen") -> [w1348]
          tunnel: w938 -> [w1318]
          shift-right: [w1314] -> _
          shift-left: w1008 -> [w1313]
          shift-right: [w1309] -> _
          shift-left: w1006 -> [w1311]
          shift-right: [w1298] -> _
          shift-left: w1006 -> [w1310]
          shift-right: ["Detektor"] -> _
          shift-left: 0 ("Detektor") -> [w1307]
          tunnel: w945 -> [w1296]
          stop <- w1354 stop-if-true
          w1319 = 0.0 ("X-Achse.Bereich:Minimum")
          n348 = Unbundle(w1296) -> ("Modul1/AI sicherer Bereich"=w1289:dbl[][], "Modul2/AI sicherer Bereich"=w1274:dbl[][], "Modul3/AI sicherer Bereich"=w1265:dbl[][], "Traps/Machs sicherer Bereich"=w1256:dbl[][], w1248:dbl[][], "Metavariablen grüner Bereich"=w1239:dbl[][])
          n349 = call "Bis zum nächsten Vielfachen warten14"("Count(mSec)"=u32 1000) -> ()  [unwired: 1 out]
          n350 = global read "GVMWHorst.vi" "MWHorst"() -> (w1247:dbl[])
          "MWHorst" <- w1247
          n351 = case shown="0, Default" "Detektor" {
            tunnel: [w1364 w1376] -> w1309
            tunnel: w1318 -> [w1363 w1378]
            tunnel: "Detektor" -> [w1358 w1372]
            tunnel: [w1362 w1377] -> w1316
            tunnel: [w1361 w1375] -> w1314
            frame 0, Default {
              n352 = Increment(x=w1358) -> (x+1=w1359:i32)
              n353 = Increment(x=w1359) -> (x+1=w1357:i32)
              n354 = global read "GVChroms.vi" "ECD1Chrom"() -> (w1360:dbl[])
              n355 = global read "GVaktuelleTDMS.vi" "aktuelleTDMS-DateiECD1"() -> (w1361:refnum<k34>)
              n356 = Index Array(array=w1363, index=w1357) -> (element=w1362:dbl)
              n357 = Array Size(array=w1360) -> (size(s)=w1366:i32)
              n358 = for {
                N: w1366 -> [_]
                tunnel: [w1367] -> w1365 mode=indexing
                i -> [w1370]
                n359 = To Double Precision Float(number=w1370) -> (double precision float=w1369:dbl)
                n360 = Divide(x=w1369, y=10.0) -> (x/y=w1367:dbl)
              }
              n361 = Bundle(w1365, "ECD1Chrom"=w1360) -> (w1364:cluster{dbl[], "ECD1Chrom":dbl[]})  [unwired: 1 in]
            }
            frame 1 {
              n362 = Increment(x=w1372) -> (x+1=w1373:i32)
              n363 = Increment(x=w1373) -> (x+1=w1371:i32)
              n364 = global read "GVChroms.vi" "ECD2Chrom"() -> (w1374:dbl[])
              n365 = global read "GVaktuelleTDMS.vi" "aktuelleTDMS-DateiECD2"() -> (w1375:refnum<k34>)
              n366 = Index Array(array=w1378, index=w1371) -> (element=w1377:dbl)
              n367 = Array Size(array=w1374) -> (size(s)=w1380:i32)
              n368 = for {
                N: w1380 -> [_]
                tunnel: [w1381] -> w1379 mode=indexing
                i -> [w1384]
                n369 = To Double Precision Float(number=w1384) -> (double precision float=w1383:dbl)
                n370 = Divide(x=w1383, y=10.0) -> (x/y=w1381:dbl)
              }
              n371 = Bundle(w1379, "ECD2Chrom"=w1374) -> (w1376:cluster{dbl[], "ECD2Chrom":dbl[]})  [unwired: 1 in]
            }
          }
          n372 = Subtract(x="DetYMax", y="DetYMin") -> (x-y=w1324:dbl)
          n373 = Subtract(x="HK1YMax", y="HK1YMin") -> (x-y=w1334:dbl)
          n374 = Subtract(x="HK2YMax", y="HK2YMin") -> (x-y=w1329:dbl)
          n375 = Equal?(x="Detektor", y=w1307) -> (x = y?=w1306:bool)
          n376 = Index Array(array=w1289, index (col) #1=0 ("disabled index (col)"), index (col) #2=1 ("index (col)")) -> (element #1=w1286:dbl[], element #2=w1284:dbl[])  [unwired: 2 in]
          n377 = Index Array(array=w1274, index (col) #1=0 ("disabled index (col)"), index (col) #2=1 ("index (col)")) -> (element #1=w1278:dbl[], element #2=w1277:dbl[])  [unwired: 2 in]
          n378 = Index Array(array=w1256, index (col) #1=0 ("disabled index (col)"), index (col) #2=1 ("index (col)")) -> (element #1=w1260:dbl[], element #2=w1259:dbl[])  [unwired: 2 in]
          n379 = Index Array(array=w1248, index (col) #1=0 ("disabled index (col)"), index (col) #2=1 ("index (col)")) -> (element #1=w1252:dbl[], element #2=w1251:dbl[])  [unwired: 2 in]
          n380 = Index Array(array=w1265, index (col) #1=0 ("disabled index (col)"), index (col) #2=1 ("index (col)")) -> (element #1=w1269:dbl[], element #2=w1268:dbl[])  [unwired: 2 in]
          n381 = Index Array(array=w1239, index (col) #1=0 ("disabled index (col)"), index (col) #2=1 ("index (col)")) -> (element #1=w1243:dbl[], element #2=w1242:dbl[])  [unwired: 2 in]
          n382 = global read "GVMethodenwechsel.vi" "Methodenwechsel?"() -> (w1352:bool)
          n383 = global read "GVZeitenZyklen.vi" "ZyklusNummern"() -> (w1321:i32[])
          "ZyklusNummern" <- w1321
          n384 = global read "gvbooleschRT.vi" "global stop RT"() -> (w1353:bool)
          n385 = global read "GVMetavariablen.vi" "Metavariablen"() -> (w1238:dbl[])
          "MVWerte" <- w1238
          n386 = global read "GVVentilposition.vi" "Ventilposition"() -> (→"Ventilposition":i32)
          n387 = global read "GVZeitenZyklen.vi" "ZyklusNummernGesamt"() -> (→"ZyklusNummernGesamt":i32[])
          n388 = call <vilib>:"RT Get CPU Loads.vi"() -> ("CPU loads"=w1232:T27[])  [unwired: 10 in, 1 out]
          n389 = Divide(x=w1324, y=20.0) -> (x/y=w1322:dbl)
          n390 = Divide(x=w1334, y=10.0) -> (x/y=w1332:dbl)
          n391 = Divide(x=w1329, y=10.0) -> (x/y=w1327:dbl)
          n392 = Index Array(array=w1232, index=0) -> (element=w1230:T27)
          n393 = local read "veränderte Methode benutzen"() -> (w1351:bool)
          n394 = Or(x=w1352, y=w1353) -> (x .or. y?=w1355:bool)
          n395 = Greater Or Equal?(x=w1247, y=w1252) -> (x >= y?=w1250:bool[])
          n396 = Less Or Equal?(x=w1247, y=w1251) -> (x <= y?=w1249:bool[])
          n397 = Greater Or Equal?(x=w1238, y=w1243) -> (x >= y?=w1241:bool[])
          n398 = Less Or Equal?(x=w1238, y=w1242) -> (x <= y?=w1240:bool[])
          n399 = Unbundle(w1230) -> ("Total (%)"=→"CPU Total (%)":dbl)  [unwired: 8 out]
          n400 = global read "GVHK1Hz.vi" "Mod1Mod2Mod3/AITrapsMachs1Hz"() -> (w1234:dbl[])
          n401 = global write "GVMetavariablen.vi" "MVFixwert"("MVFixwert") -> ()
          n402 = And(x=w1250, y=w1249) -> (x .and. y?=→"HorstOK?":bool[])
          n403 = And(x=w1241, y=w1240) -> (x .and. y?=→"MVOK?":bool[])
          n404 = Or(x=w1355, y=w1351) -> (x .or. y?=w1354:bool)
          n405 = global write "GVMetavariablen.vi" "MVFix?"("MVFix?") -> ()
          n406 = global read "GVZeitenZyklen.vi" "Big Ben, Methodenzeit, Zykluszeit0, Zykluszeit1, Zykluszeit2A, Zykluszeit2B"() -> (w1301:dbl[])
          n407 = Array Subset(array=w1234, index=0 ("Index"), length=32 ("Länge")) -> (w1285:dbl[])
          "AIs1" <- w1285
          n408 = Array Subset(array=w1234, index=32 ("Index"), length=32 ("Länge")) -> (w1273:dbl[])
          "AIs2" <- w1273
          n409 = Array Subset(array=w1234, index=96 ("Index"), length=6 ("Länge")) -> (w1233:dbl[])
          "schnelle Heizungen" <- w1233
          n410 = Array Subset(array=w1234, index=64 ("Index"), length=32 ("Länge")) -> (w1264:dbl[])
          "AIs3" <- w1264
          n411 = Greater Or Equal?(x=w1233, y=w1260) -> (x >= y?=w1258:bool[])
          n412 = Less Or Equal?(x=w1233, y=w1259) -> (x <= y?=w1257:bool[])
          n413 = Greater Or Equal?(x=w1285, y=w1286) -> (x >= y?=w1283:bool[])
          n414 = Less Or Equal?(x=w1285, y=w1284) -> (x <= y?=w1282:bool[])
          n415 = Greater Or Equal?(x=w1273, y=w1278) -> (x >= y?=w1276:bool[])
          n416 = Less Or Equal?(x=w1273, y=w1277) -> (x <= y?=w1275:bool[])
          n417 = And(x=w1258, y=w1257) -> (x .and. y?=→"SHOK?":bool[])
          n418 = Greater Or Equal?(x=w1264, y=w1269) -> (x >= y?=w1267:bool[])
          n419 = Less Or Equal?(x=w1264, y=w1268) -> (x <= y?=w1266:bool[])
          n420 = And(x=w1283, y=w1282) -> (x .and. y?=→"AIs1OK?":bool[])
          n421 = And(x=w1276, y=w1275) -> (x .and. y?=→"AIs2OK?":bool[])
          n422 = And(x=w1267, y=w1266) -> (x .and. y?=→"AIs3OK?":bool[])
          n423 = To Long Integer(number=w1301) -> (32bit integer=→"Big Ben, Methodenzeit, Zykluszeit0, Zykluszeit1, Zykluszeit2A, Zykluszeit2B":i32[])
          n424 = Equal?(x=w1314, y=w1313) -> (x = y?=w1312:bool)
          n425 = call "AnzeigeGV.vi"("veränderte Methode benutzen"=w1351, "Zykluslängen [s]"=w1318, "Cluster1"=w1350, "Big Ben, Methodenzeit, Zykluszeit0, Zykluszeit1, Zykluszeit2A, Zykluszeit2B"=w1301, "Zyklusnummern 0, 1, 2A, 2B"=w1321, "Cluster2"=w1349, "AnzeigeEinstellungen"=w1348, "dargestellte Größe 1"="dargestellte Größe 1", "Zeitachse1"="Zeitachse1", "dargestellte Größe 2"="dargestellte Größe 2", "Zeitachse2"="Zeitachse2") -> ("Anzeige2"=→"Housekeeping2":cluster{dbl[], dbl[]}, "Cluster1"=w1343:cluster{dbl[], dbl[], dbl[], dbl[]}, "x1Inkr"=w1338:dbl, "Cluster2"=w1342:cluster{dbl[], dbl[], dbl[], dbl[]}, "Anzeige1"=→"Housekeeping1":cluster{dbl[], dbl[]}, "AnzeigeEinstellungen"=w1340:T16, "x2Max"=w1302:dbl, "x2Inkr"=w1337:dbl, "x1Max"=w1303:dbl)  [unwired: 8 in]
          n426 = Divide(x=w1316, y=20.0) -> (x/y=w1317:dbl)
          n427 = property on="Detektor 2" class="XYGraph (strict)"("XScale.Minimum"=w1319, "XScale.Maximum"=w1316, "XScale.Increment"=w1317, "YScale.Minimum"="DetYMin", "YScale.Maximum"="DetYMax", "YScale.Increment"=w1322) -> ()  [unwired: 2 in, 2 out]
          n428 = property on="Housekeeping1" class="XYGraph (strict)"("XScale.Minimum"=w1319, "XScale.Maximum"=w1303, "XScale.Increment"=w1338, "YScale.Minimum"="HK1YMin", "YScale.Maximum"="HK1YMax", "YScale.Increment"=w1332) -> ()  [unwired: 2 in, 2 out]
          n429 = property on="Housekeeping2" class="XYGraph (strict)"("XScale.Minimum"=w1319, "XScale.Maximum"=w1302, "XScale.Increment"=w1337, "YScale.Minimum"="HK2YMin", "YScale.Maximum"="HK2YMax", "YScale.Increment"=w1327) -> ()  [unwired: 2 in, 2 out]
          n430 = Select(t=w1310, s=w1312, f=w1311) -> (s? t:f=w1305:cluster{dbl[], dbl[]})
          n431 = Select(t=w1305, s=w1306, f=cluster{dbl[], dbl[]} {[], []} ("s? t:f")) -> (s? t:f=w1298:cluster{dbl[], dbl[]})
          n432 = Build Array(w1309, w1298) -> (→"Detektor 2":cluster{dbl[], "ECD2Chrom":dbl[]}[])
        }
        n433 = while "ZyklusSteuerung" {
          tunnel: w1043 -> [w1388]
          tunnel: w1044 -> [w1394]
          shift-right: [w1386] -> _
          shift-left: w1018 -> [w1392]
          tunnel: w1026 -> [w1393]
          tunnel: w944 -> [w1389]
          tunnel: w943 -> [w1390]
          tunnel: w942 -> [w1391]
          shift-right: [w1385] -> _
          shift-left: errorcluster {"status"=FALSE, "code"=0, "source"=""} ("error out") -> [w1387]
          stop <- w1395 stop-if-true
          n434 = call "Bis zum nächsten Vielfachen warten11"("Count(mSec)"=u32 100) -> ()  [unwired: 1 out]
          n435 = global read "GVMethodenwechsel.vi" "Methodenwechsel?"() -> (w1398:bool)
          n436 = global read "gvbooleschRT.vi" "global stop RT"() -> (w1397:bool)
          n437 = local read "veränderte Methode benutzen"() -> (w1396:bool)
          n438 = Compound Arithmetic op=OR(w1398, w1397, w1396) -> (w1395:bool)
          n439 = call "ZyklussteuerungGV-15-07-17.vi"("Traps/MachKoeff0"=w1389, "DIOsNummern"=w1388, "error in"=w1387, "Traps/MachKoeff1"=w1390, "Traps/MachKoeff2"=w1391, "Schieberegister"=w1392, "Zeitpunkte/Setpoints"=w1393, "FPGA VI Reference In"=w1394) -> ("Schieberegister"=w1386:T28, "error out"=w1385:errorcluster)  [unwired: 6 in]
          "Zyklus" <- w1385
        }
        n440 = global read "GVZeitenZyklen.vi" "Big Ben, Methodenzeit, Zykluszeit0, Zykluszeit1, Zykluszeit2A, Zykluszeit2B"() -> (w1005:dbl[])
        n441 = Index Array(array=w1005, index=3 ("Index")) -> (element=w1003:dbl)
        n442 = while {
          tunnel: w1047 -> [w1171]
          tunnel: w1046 -> [w1170]
          tunnel: w969 -> [w1185]
          shift-right: [w1186] -> w1040
          shift-left: w1045 -> [w1187]
          tunnel: w966 -> [w1181]
          tunnel: w965 -> [w1175]
          shift-right: [w1172] -> _
          shift-left: w1003 -> [w1176]
          stop <- w1188 stop-if-true
          n443 = Less?(x=w1176, y=w1181) -> (x < y?=w1179:bool)
          n444 = Less?(x=w1176, y=w1175) -> (x < y?=w1177:bool)
          n445 = call "Bis zum nächsten Vielfachen warten13"("Count(mSec)"=u32 100 ("Zu wartende ms")) -> ()  [unwired: 1 out]
          n446 = global read "GVMethodenwechsel.vi" "Methodenwechsel?"() -> (w1190:bool)
          n447 = global read "gvbooleschRT.vi" "global stop RT"() -> (w1191:bool)
          n448 = local read "veränderte Methode benutzen"() -> (w1189:bool)
          n449 = Compound Arithmetic op=OR(w1191, w1190, w1189) -> (w1188:bool)
          n450 = global read "GVZeitenZyklen.vi" "Big Ben, Methodenzeit, Zykluszeit0, Zykluszeit1, Zykluszeit2A, Zykluszeit2B"() -> (w1183:dbl[])
          n451 = Index Array(array=w1183, index=3 ("Index")) -> (element=w1172:dbl)
          n452 = Greater Or Equal?(x=w1172, y=w1181) -> (x >= y?=w1180:bool)
          n453 = Greater Or Equal?(x=w1172, y=w1175) -> (x >= y?=w1178:bool)
          n454 = And(x=w1178, y=w1177) -> (x .and. y?=w1174:bool)
          n455 = And(x=w1180, y=w1179) -> (x .and. y?=w1169:bool)
          n456 = Or(x=w1169, y=w1174) -> (x .or. y?=w1173:bool)
          n457 = And(x=w1185, y=w1173) -> (x .and. y?=w1184:bool)
          n458 = case shown="True" w1184 {
            tunnel: w1187 -> [w1193 w1194]
            tunnel: [w1193 w1198] -> w1186
            tunnel: w1171 -> [_ w1197]
            tunnel: w1170 -> [_ w1196]
            tunnel: w1169 -> [_ w1195]
            frame False {
            }
            frame True {
              n459 = call "MSDateienSchicken12-15.vi"("MSNummer"=w1194, "MSa?"=w1195, "Dateipfad:fromcriordy"=w1196, "Dateipfad:fromcriocmd"=w1197) -> ()  [unwired: 1 in]
              n460 = Increment(x=w1194) -> (x+1=w1198:i32)
            }
          }
        }
      }
      n461 = case shown="True" TRUE ("HKSpeichern") {
        tunnel: w549 -> [_ w914]
        frame False {
        }
        frame True {
          n462 = while {
            tunnel: w914 -> [w918]
            shift-right: [w916] -> _
            shift-left: errorcluster {"status"=FALSE, "code"=0, "source"=""} ("error out") -> [w915]
            stop <- w920 stop-if-true
            n463 = call "Bis zum nächsten Vielfachen warten2"("Count(mSec)"=u32 1000) -> ()  [unwired: 1 out]
            n464 = local read "Methode"() -> (w917:i32)
            n465 = global read "gvbooleschRT.vi" "global stop RT"() -> (w920:bool)
            n466 = call "HKinTDMS-01-16.vi"("Methode"=w917, "error in (no error)"=w915, "Kanäle"=w918) -> ("error out"=w916:errorcluster)
            "TDMSwriteHK" <- w916
          }
        }
      }
      n467 = Concatenate Strings("?SE0,GDATA" ("Schreibpuffer"), "\r") -> (w455:string)
      n468 = Build Array(w514, w513, w512) -> (w511:i32[])
      n469 = Add Array Elements(numeric array=w511) -> (sum=w521:i32)
      n470 = Index Array(array=w511, index #1=0 ("Index"), index #2=1 ("Index")) -> (element #1=w532:i32, element #2=w530:i32)
      n471 = while {
        stop <- w1460 stop-if-true
        w1454 = 10.0
        n472 = call "Warten2"("Count(mSec)"=u32 1000) -> ()  [unwired: 1 out]
        n473 = global read "gvbooleschRT.vi" "global stop RT"() -> (w1460:bool)
        n474 = global read "GVTrapsMachs.vi" "Traps/Machs"() -> (w1450:dbl[])
        n475 = global read "GVAIs.vi" "AIs"() -> (w1451:dbl[])
        n476 = for {
          N: 9 -> [_]
          shift-right: [w1463] -> w1457
          shift-left: w1451 -> [w1464]
          shift-right: [w1461] -> w1455
          shift-left: w1450 -> [w1462]
          n477 = flat-sequence {
            tunnel: w1464 -> [w1471]
            tunnel: [w1470] -> w1463
            tunnel: w1462 -> [w1469]
            tunnel: [w1468] -> w1461
            frame #0 {
              n478 = call "Warten28"("Count(mSec)"=u32 100) -> ()  [unwired: 1 out]
            }
            frame #1 {
              n479 = global read "GVAIs.vi" "AIs"() -> (w1467:dbl[])
              n480 = Add(x=w1471, y=w1467) -> (x+y=w1470:dbl[])
              n481 = global read "GVTrapsMachs.vi" "Traps/Machs"() -> (w1466:dbl[])
              n482 = Add(x=w1466, y=w1469) -> (x+y=w1468:dbl[])
            }
          }
        }
        n483 = Divide(x=w1457, y=w1454) -> (x/y=w1456:dbl[])
        n484 = Divide(x=w1455, y=w1454) -> (x/y=w1453:dbl[])
        n485 = Build Array (concatenate)(w1456, w1453) -> (w1452:dbl[])
        n486 = global write "GVHK1Hz.vi" "Mod1Mod2Mod3/AITrapsMachs1Hz"(w1452) -> ()
      }
      n487 = Split 1D Array(array=w510, index=w532) -> (first subarray=w536:dbl[], second subarray=w540:dbl[])
      n488 = Split 1D Array(array=w508, index=w532) -> (first subarray=w539:string[], second subarray=w541:string[])
      n489 = Split 1D Array(array=w509, index=w532) -> (first subarray=w529:string[], second subarray=w531:string[])
      n490 = Initialize Array(-1.0 ("Element"), w521) -> (w506:dbl[])
      n491 = case shown="True" TRUE ("ECDSpeichern") {
        frame False {
        }
        frame True {
          w861 = dbl[] []
          n492 = global read "GVaktuelleTDMS.vi" "aktuelleTDMS-DateiECD1"() -> (w862:refnum<k34>)
          n493 = while {
            shift-right: [w874] -> _
            shift-left: w861 -> [w878]
            shift-right: [w867] -> _
            shift-left: w861 -> [w871]
            shift-right: [w873] -> _
            shift-left: w862 -> [w876]
            tunnel: w861 -> [w870]
            shift-right: [w864] -> _
            shift-left: errorcluster {"status"=FALSE, "code"=0, "source"=""} ("error IO") -> [w863]
            stop <- w883 stop-if-true
            n494 = call "Bis zum nächsten Vielfachen warten3"("Count(mSec)"=u32 500) -> ()  [unwired: 1 out]
            n495 = global read "GVECDs.vi" "ECD1MW"() -> (w877:dbl[])
            n496 = global read "GVECDs.vi" "ECD2MW"() -> (w868:dbl[])
            n497 = global read "gvbooleschRT.vi" "global stop RT"() -> (w883:bool)
            n498 = Build Array (concatenate)(w878, w877) -> (w875:dbl[])
            n499 = Build Array (concatenate)(w871, w868) -> (w872:dbl[])
            n500 = global read "GVaktuelleTDMS.vi" "aktuelleTDMS-DateiECD1"() -> (w873:refnum<k34>)
            n501 = global read "GVaktuelleTDMS.vi" "aktuelleTDMS-DateiECD2"() -> (w881:refnum<k34>)
            n502 = Equal?(x=w876, y=w873) -> (x = y?=w869:bool)
            n503 = TDMS Write(0:w873, 7:"ECD1", 9:w877, 11:w863) -> (15:w866:errorcluster)  [unwired: 2 in, 3 out]
            n504 = TDMS Write(0:w881, 7:"ECD2", 9:w868, 11:w863) -> (15:w865:errorcluster)  [unwired: 2 in, 3 out]
            n505 = Select(t=w875, s=w869, f=w870) -> (s? t:f=w874:dbl[])
            n506 = Select(t=w872, s=w869, f=w870) -> (s? t:f=w867:dbl[])
            n507 = global write "GVChroms.vi" "ECD1Chrom"(w874) -> ()
            n508 = global write "GVChroms.vi" "ECD2Chrom"(w867) -> ()
            n509 = Merge Errors(w866, w865) -> (w864:errorcluster)
            "TDMSwriteECD" <- w864
          }
        }
      }
      n510 = while {
        shift-right: [w558] -> _
        shift-left: w454 -> [w560]
        shift-right: [w557] -> _
        shift-left: w454 -> [w559]
        stop <- w562 stop-if-true
        n511 = call "Bis zum nächsten Vielfachen warten"("Count(mSec)"=u32 100) -> ()  [unwired: 1 out]
        n512 = case shown="True" "An/Aus" {
          tunnel: w560 -> [w564 w580]
          tunnel: w559 -> [w563 w579]
          tunnel: [w564 w573] -> w558
          tunnel: [w563 w572] -> w557
          frame False {
          }
          frame True {
            w576 = dbl[] [] ("t")
            n513 = global read "GVMWHorst.vi" "MWHorst"() -> (w569:dbl[])
            n514 = global read "GVTrapsMachs.vi" "Traps/Machs"() -> (w570:dbl[])
            n515 = Build Array (concatenate)(w570, w569) -> (w568:dbl[])
            n516 = Index Array(array=w568, index="dargestellte Größe 3") -> (element=w581:dbl)
            n517 = Build Array (concatenate)(w580, w581) -> (w574:dbl[])
            n518 = Select(t=w576, s="TafelWischen!", f=w574) -> (s? t:f=w573:dbl[])
            n519 = global read "GVZeitenZyklen.vi" "Big Ben, Methodenzeit, Zykluszeit0, Zykluszeit1, Zykluszeit2A, Zykluszeit2B"() -> (w567:dbl[])
            n520 = Index Array(array=w567, index=1 ("Index")) -> (element=w565:dbl)
            n521 = Build Array (concatenate)(w579, w565) -> (w575:dbl[])
            n522 = Select(t=w576, s="TafelWischen!", f=w575) -> (s? t:f=w572:dbl[])
            n523 = Bundle(w575, w574) -> (→"schnelleAnzeige":cluster{dbl[], dbl[]})  [unwired: 1 in]
          }
        }
        n524 = global read "gvbooleschRT.vi" "global stop RT"() -> (w562:bool)
      }
      n525 = case shown="True" TRUE {
        tunnel: w500 -> [_ w893]
        tunnel: w498 -> [_ w892]
        tunnel: w497 -> [_ w891]
        tunnel: w492 -> [_ w890]
        tunnel: w491 -> [_ w889]
        frame False {
        }
        frame True {
          w884 = errorcluster {"status"=FALSE, "code"=0, "source"=""} ("error out TDMSopen")
          n526 = while {
            shift-right: [w898] -> w888
            shift-left: w890 -> [w900]
            shift-right: [w909] -> w887
            shift-left: w889 -> [w902]
            shift-right: [w904] -> _
            shift-left: w893 -> [w910]
            tunnel: w891 -> [w906]
            tunnel: w892 -> [w907]
            shift-right: [w897] -> w886
            shift-left: w884 -> [w895]
            shift-right: [w896] -> w885
            shift-left: w884 -> [w894]
            stop <- w912 stop-if-true
            n527 = call "Bis zum nächsten Vielfachen warten5"("Count(mSec)"=u32 500) -> ()  [unwired: 1 out]
            n528 = local read "Methode"() -> (w908:i32)
            n529 = global read "gvbooleschRT.vi" "global stop RT"() -> (w912:bool)
            n530 = global read "GVZeitenZyklen.vi" "ZyklusNummernGesamt"() -> (w899:i32[])
            n531 = Index Array(array=w899, index=1 ("Index")) -> (element=w904:i32)
            n532 = Greater?(x=w904, y=w910) -> (0:w903:bool)
            n533 = Select(t=w902, s=w903, f=w900) -> (s? t:f=w901:refnum<k34>)
            n534 = call "AktuelleTDMS.vi"("AktuelleTDMS"=w900, "error in TDMSopen"=w895, "Dateiordner"=w907, "NächsteTDMS"=w902, "NeuerZyklus?"=w903, "Methodennummer"=w908, "Zyklnumges"=w904, "error in TDMSclose"=w894, "Dateiname"=w906) -> ("AktuelleTDMS"=w898:refnum<k34>, "error out TDMSopen"=w897:errorcluster, "error out TDMSclose"=w896:errorcluster, "NächsteTDMS"=w909:refnum<k34>)  [unwired: 3 in]
            "TDMSopenHK" <- w897
            "TDMScloseHK" <- w896
            n535 = global write "GVaktuelleTDMS.vi" "aktuelleTDMS-DateiHK"(w901) -> ()
          }
          n536 = TDMS Close(8:w886, 11:w888) -> ()  [unwired: 2 out]
          n537 = TDMS Close(8:w885, 11:w887) -> ()  [unwired: 2 out]
        }
      }
      n538 = case shown="True" TRUE {
        tunnel: w500 -> [_ w821]
        tunnel: w496 -> [_ w820]
        tunnel: w495 -> [_ w819]
        tunnel: w494 -> [_ w818]
        tunnel: w493 -> [_ w817]
        tunnel: w490 -> [_ w816]
        tunnel: w489 -> [_ w815]
        tunnel: w488 -> [_ w814]
        tunnel: w487 -> [_ w813]
        frame False {
        }
        frame True {
          w806 = errorcluster {"status"=FALSE, "code"=0, "source"=""} ("error out TDMSopen")
          n539 = while {
            shift-right: [w845] -> w812
            shift-left: w816 -> [w847]
            shift-right: [w855] -> w811
            shift-left: w815 -> [w849]
            shift-right: [w853] -> _
            shift-left: w821 -> [w856]
            tunnel: w820 -> [w852]
            tunnel: w818 -> [w851]
            shift-right: [w844] -> w807
            shift-left: w806 -> [w842]
            shift-right: [w843] -> w808
            shift-left: w806 -> [w841]
            stop <- w858 stop-if-true
            n540 = call "Bis zum nächsten Vielfachen warten4"("Count(mSec)"=u32 500) -> ()  [unwired: 1 out]
            n541 = local read "Methode"() -> (w854:i32)
            n542 = global read "gvbooleschRT.vi" "global stop RT"() -> (w858:bool)
            n543 = global read "GVZeitenZyklen.vi" "ZyklusNummernGesamt"() -> (w846:i32[])
            n544 = Index Array(array=w846, index=2 ("Index")) -> (element=w853:i32)
            n545 = Greater?(x=w853, y=w856) -> (0:w850:bool)
            n546 = Select(t=w849, s=w850, f=w847) -> (s? t:f=w848:refnum<k34>)
            n547 = call "AktuelleTDMS.vi"("AktuelleTDMS"=w847, "error in TDMSopen"=w842, "Dateiordner"=w852, "NächsteTDMS"=w849, "NeuerZyklus?"=w850, "Methodennummer"=w854, "Zyklnumges"=w853, "error in TDMSclose"=w841, "Dateiname"=w851) -> ("AktuelleTDMS"=w845:refnum<k34>, "error out TDMSopen"=w844:errorcluster, "error out TDMSclose"=w843:errorcluster, "NächsteTDMS"=w855:refnum<k34>)  [unwired: 3 in]
            "TDMSopenECD1" <- w844
            "TDMScloseECD1" <- w843
            n548 = global write "GVaktuelleTDMS.vi" "aktuelleTDMS-DateiECD1"(w848) -> ()
          }
          n549 = while {
            shift-right: [w835] -> w810
            shift-left: w814 -> [w827]
            shift-right: [w836] -> w809
            shift-left: w813 -> [w829]
            shift-right: [w833] -> _
            shift-left: w821 -> [w837]
            tunnel: w819 -> [w832]
            tunnel: w817 -> [w831]
            shift-right: [w825] -> _
            shift-left: w806 -> [w823]
            shift-right: [w824] -> _
            shift-left: w806 -> [w822]
            stop <- w839 stop-if-true
            n550 = call "Bis zum nächsten Vielfachen warten6"("Count(mSec)"=u32 500) -> ()  [unwired: 1 out]
            n551 = local read "Methode"() -> (w834:i32)
            n552 = global read "gvbooleschRT.vi" "global stop RT"() -> (w839:bool)
            n553 = global read "GVZeitenZyklen.vi" "ZyklusNummernGesamt"() -> (w826:i32[])
            n554 = Index Array(array=w826, index=3 ("Index")) -> (element=w833:i32)
            n555 = Greater?(x=w833, y=w837) -> (0:w830:bool)
            n556 = Select(t=w829, s=w830, f=w827) -> (s? t:f=w828:refnum<k34>)
            n557 = call "AktuelleTDMS.vi"("AktuelleTDMS"=w827, "error in TDMSopen"=w823, "Dateiordner"=w832, "NächsteTDMS"=w829, "NeuerZyklus?"=w830, "Methodennummer"=w834, "Zyklnumges"=w833, "error in TDMSclose"=w822, "Dateiname"=w831) -> ("AktuelleTDMS"=w835:refnum<k34>, "error out TDMSopen"=w825:errorcluster, "error out TDMSclose"=w824:errorcluster, "NächsteTDMS"=w836:refnum<k34>)  [unwired: 3 in]
            "TDMSopenECD2" <- w825
            "TDMScloseECD2" <- w824
            n558 = global write "GVaktuelleTDMS.vi" "aktuelleTDMS-DateiECD2"(w828) -> ()
          }
          n559 = TDMS Close(8:w807, 11:w812) -> ()  [unwired: 2 out]
          n560 = TDMS Close(8:w808, 11:w811) -> ()  [unwired: 2 out]
          n561 = TDMS Close(11:w810) -> ()  [unwired: 1 in, 2 out]
          n562 = TDMS Close(11:w809) -> ()  [unwired: 1 in, 2 out]
        }
      }
      n563 = Split 1D Array(array=w541, index=w530) -> (first subarray=w538:string[], second subarray=w537:string[])
      n564 = Split 1D Array(array=w540, index=w530) -> (first subarray=w535:dbl[], second subarray=w534:dbl[])
      n565 = Split 1D Array(array=w531, index=w530) -> (first subarray=w528:string[], second subarray=w527:string[])
      n566 = Bundle(w539, w538, w537, w536, w535, w534) -> (w533:T29)  [unwired: 1 in]
      n567 = Bundle(w529, w528, w527) -> (w526:cluster{string[], string[], string[]})  [unwired: 1 in]
      n568 = Initialize Array(0.0, 8 ("Dimension")) -> (w456:dbl[])
      n569 = Bundle(w525, w525, w525) -> (w524:cluster{i32, i32, i32})  [unwired: 1 in]
      n570 = Initialize Array("x", 8 ("Dimension")) -> (w461:string[])
      n571 = case shown="True" TRUE ("SerielleKomm.") {
        tunnel: bool[] [TRUE, TRUE, TRUE, TRUE, TRUE, TRUE, TRUE, TRUE] -> [_ w598]
        tunnel: w461 -> [_ w597]
        tunnel: w533 -> [_ w596]
        tunnel: w532 -> [_ w595]
        tunnel: w530 -> [_ w594]
        tunnel: w526 -> [_ w593]
        tunnel: w524 -> [_ w592]
        tunnel: w523 -> [_ w591]
        tunnel: w510 -> [_ w590]
        tunnel: w507 -> [_ w589]
        tunnel: w506 -> [_ w588]
        tunnel: w505 -> [_ w585]
        tunnel: w484 -> [_ w587]
        tunnel: w456 -> [_ w586]
        tunnel: w455 -> [_ w584]
        frame False {
        }
        frame True {
          n572 = while {
            tunnel: w585 -> [w612]
            tunnel: w584 -> [w611]
            shift-right: [w610] -> _
            shift-left: errorcluster {"status"=FALSE, "code"=0, "source"=""} ("error out") -> [w609]
            stop <- w613 stop-if-true
            n573 = call "Warten6"("Count(mSec)"=u32 500) -> ()  [unwired: 1 out]
            n574 = global read "gvbooleschRT.vi" "global stop RT"() -> (w613:bool)
            n575 = case shown="True" "NeuerRefstrom" {
              tunnel: w611 -> [w615 _]
              tunnel: [w614 w624] -> w604
              tunnel: [w614 w627] -> w600
              frame False {
                n576 = String To Byte Array(string=w615) -> (unsigned byte array=w614:u8[])
              }
              frame True {
                n577 = local write "NeuerRefstrom"(FALSE ("NeuerRefstrom")) -> ()
                n578 = Number To Decimal String(number="RefStromECD1", width (-)=i16 4) -> (decimal integer string=w619:string)
                n579 = Number To Decimal String(number="RefStromECD2", width (-)=i16 4) -> (decimal integer string=w616:string)
                n580 = Concatenate Strings("?SE0,SETP," ("string"), w619, "\r\n") -> (w628:string)
                n581 = Concatenate Strings("?SE0,SETP," ("string"), w616, "\r\n") -> (w625:string)
                n582 = String To Byte Array(string=w628) -> (unsigned byte array=w627:u8[])
                n583 = String To Byte Array(string=w625) -> (unsigned byte array=w624:u8[])
              }
            }
            n584 = Join Numbers(hi=w600, lo=u8 5) -> ((hi.lo)=w606:u16[])
            n585 = Join Numbers(hi=w604, lo=u8 6) -> ((hi.lo)=w602:u16[])
            n586 = xnode "Invoke Method"("FPGA VI Reference In"=w612, "error in"=w609, "Data"=w606) -> ("FPGA VI Reference Out"=w605:refnum<k20>, "error out"=w601:errorcluster)  [unwired: 1 in, 1 out]
            n587 = xnode "Invoke Method"("FPGA VI Reference In"=w605, "error in"=w601, "Data"=w602) -> ("error out"=w610:errorcluster)  [unwired: 1 in, 2 out]
            "FIFOwriteRS485" <- w610
          }
          n588 = while {
            shift-right: [w763] -> _
            shift-left: w598 -> [w783]
            shift-right: [w787] -> _
            shift-left: w588 -> [w793]
            tunnel: w585 -> [w780]
            shift-right: [w764] -> _
            shift-left: w597 -> [w768]
            tunnel: w589 -> [w771]
            tunnel: w590 -> [w766]
            shift-right: [w772] -> _
            shift-left: w591 -> [w789]
            tunnel: w595 -> [w791]
            tunnel: w594 -> [w792]
            tunnel: w596 -> [w794]
            tunnel: w593 -> [w777]
            shift-right: [w773] -> _
            shift-left: w592 -> [w776]
            shift-right: [w779] -> _
            shift-left: w587 -> [w782]
            shift-right: [w784] -> _
            shift-left: w586 -> [w785]
            shift-right: [w765] -> _
            shift-left: errorcluster {"status"=FALSE, "code"=0, "source"=""} ("error out") -> [w781]
            stop <- w788 stop-if-true
            n589 = for {
              tunnel: w783 -> [w798] mode=indexing
              tunnel: w785 -> [w795] mode=indexing
              tunnel: [w802] -> w784 mode=indexing
              tunnel: [w799] -> w775 mode=indexing
              n590 = global read "GVZeitenZyklen.vi" "Big Ben, Methodenzeit, Zykluszeit0, Zykluszeit1, Zykluszeit2A, Zykluszeit2B"() -> (w805:dbl[])
              n591 = Index Array(array=w805, index=0 ("Index")) -> (element=w803:dbl)
              n592 = Subtract(x=w803, y=w795) -> (x-y=w801:dbl)
              n593 = Greater?(x=w801, y=0.1) -> (0:w797:bool)
              n594 = Or(x=w798, y=w797) -> (x .or. y?=w796:bool)
              n595 = Select(t=w797, s=w797, f=w798) -> (s? t:f=w799:bool)
              n596 = Select(t=w803, s=w796, f=w795) -> (s? t:f=w802:dbl)
            }
            n597 = global read "GVHorstSP.vi" "HorstSP"() -> (w787:dbl[])
            n598 = Not Equal?(x=w787, y=w793) -> (x != y?=w790:bool)
            n599 = call "NeueSP.vi"("Anzahl2"=w792, "Anzahl1"=w791, "AlteSP"=w793, 7:"NeueSP"=w787, "BefehleCluster"=w789, 10:"NeueSP"=w790, "ClusterFest"=w794) -> ("BefehleCluster"=w774:T30)  [unwired: 4 in]
            n600 = call "Warten3"("Count(mSec)"=u32 50) -> ()  [unwired: 1 out]
            n601 = call "MPVSenden-15-07-17.vi"("Ventilposition"=w782, "error in"=w781, "FPGA VI Reference In"=w780) -> ("Ventilposition"=w779:i32, "error out"=w778:errorcluster, "FPGA VI Reference Out"=w770:refnum<k20>)
            n602 = call "Senden-15-07-17.vi"("error in"=w778, "BefehlsCluster"=w774, "AbfragenCluster"=w777, "Abfragenr.Cluster"=w776, "Senden?"=w775, "FPGA VI Reference In"=w770) -> ("BefehlsCluster"=w772:T30, "error out"=w767:errorcluster, "Senden?"=w769:bool[], "Abfragenr.Cluster"=w773:cluster{i32, i32, i32})  [unwired: 1 in]
            n603 = call "SeriellRead-15-07-17.vi"("SkalierungsfaktorHorst"=w766, "VorwortHorst"=w771, "error in"=w767, "Zwischenspeicher"=w768, "Senden?"=w769, "FPGA VI Reference In"=w770) -> ("Senden?"=w763:bool[], "Zwischenspeicher"=w764:string[], "error out"=w765:errorcluster)  [unwired: 3 in]
            "SerielleKomm." <- w765
            n604 = global read "gvbooleschRT.vi" "global stop RT"() -> (w788:bool)
          }
        }
      }
    }
    frame #2 {
      n605 = xnode "Read/Write Control"("FPGA VI Reference In"=w1479, "global stop"=TRUE) -> ("FPGA VI Reference Out"=w1478:refnum<k20>)  [unwired: 1 in, 1 out]
      n606 = xnode "Close FPGA VI Reference"("FPGA VI Reference In"=w1478) -> ()  [unwired: 1 in, 1 out]
    }
    frame #3 {
    }
    frame #4 {
    }
  }
